vi "DAQLinescan.vi"() -> ()   [LabVIEW 2009]
uses:
  ImageSettings.ctt
  DisplaySettings.ctt
  Instance          51 19Saved   DAQLinescan .vi
  Instance          52 19Saved   DAQLinescan .vi
  <vilib>/Utility/inputDevices.llb/mouseAcquire.vi
  AO Update Channel.vi
panel:
  out "Position":dbl[](array[numeric]) format="%.6f"
  in  "show position (PI digital)":bool
  in  "mouse wheel\nfocus control":bool
  out "mouse focus":cluster{"device ID":refnum<k1>, "Scrolling":i32}
  in  "Laser 4":bool
  in  "SyncTime(ns)":dbl=12.5
  in  "Laser 3":bool
  in  "Laser 2":bool
  in  "Laser 1":bool
  in  "AOTF":u16(ring) items=["None", "Laser 1", "Laser 2", "Laser 1 + 2", "Laser 3", "Laser 1 + 3", "Laser 2 + 3", "Laser 1+2+3", "Laser 1+2+3+4", "Laser 2+3+4"]
  in  "AOTF Setup":bool
  in  "x-scale: Time?":bool
  in  "Autoscale y-axis":bool=TRUE
  in  "Store Data":bool
  in  "Pick & Destroy":bool caption="stop"
  in  "Load Image":bool caption="stop"
  in  "Position Increment (µm)":cluster{"x":dbl, "y":dbl, "z":dbl}={"x"=0.1, "y"=0.1, "z"=0.1} {"z" format="%.2f"; "y" format="%.2f"; "x" format="%.2f"}
  in  "Current Position (µm)":cluster{"x":dbl, "y":dbl, "z":dbl} {"z" format="%.2f"; "y" format="%.2f"; "x" format="%.2f"}
  in  "Down (z)":bool
  in  "Up (z)":bool
  in  "Down":bool
  in  "Up":bool
  in  "Right":bool
  in  "Left":bool
  in  "Display Settings":T1={"Show MCS"=TRUE, "Show Image"=TRUE, "Color coding"=1, "Plane"=0, "Threshold"={"max"=150, "min"=0}} {"Plane" max=0; "Color coding" items=["Color Gradient", "False Color"]}
  in  "Destination:":path
  in  "Exit":bool caption="stop"
  in  "Save & Exit":bool caption="stop"
  in  "Stage Setup":bool
  in  "SPC Setup":bool
  in  "Scan":bool
  in  "EOM Setup":bool
  in  "Keep Start Position":bool=TRUE
  in  "Isotropy (x/y)":bool=TRUE
  in  "Keep Image Size":bool=TRUE
  in  "EOM":u16(ring) items=["None", "Trace", "Retrace", "All"]
  in  "Read Position":bool
  in  "Image Settings":T2={"Start Position (µm)"={"x"=0.0, "y"=0.0, "z"=0.0}, "End Position (µm)"={"x"=10.0, "y"=10.0, "z"=10.0}, "Image Resolution (nm/pixel)"={"x"=50.0, "y"=50.0, "z"=100.0}, "Image Size (µm)"={"x"=10.0, "y"=10.0, "z"=0.0}, "Image Size (pixel)"={"x"=200, "y"=200, "z"=0}, "Time Resolution\n(ms/pixel)"=1.0, "1st Axis"=0, "2nd Axis"=1, "Retrace"=FALSE, "Estimated Time"="00:00:40"} {"2nd Axis" items=["x", "y", "z"]; "1st Axis" items=["x", "y", "z"]; "Time Resolution\n(ms/pixel)" format="%.2f"; "Image Resolution (nm/pixel)"."z" format="%.2f"; "Image Resolution (nm/pixel)"."y" format="%.2f"; "Image Resolution (nm/pixel)"."x" format="%.2f"; "Image Size (µm)"."z" format="%.2f"; "Image Size (µm)"."y" format="%.2f"; "Image Size (µm)"."x" format="%.2f"; "End Position (µm)"."z" format="%.2f"; "End Position (µm)"."y" format="%.2f"; "End Position (µm)"."x" format="%.2f"; "Start Position (µm)"."z" format="%.2f"; "Start Position (µm)"."y" format="%.2f"; "Start Position (µm)"."x" format="%.2f"}
  out "MCS Trace":u32[][](graph)=[[5, 9, 9, 4, 5, 7, 7, 7, 4, 6, 5, 11, 11, 6, 8, 9, 8, 5, 6, 8, 5, 5, 8, 5, 6, 5, 4, 9, 6, 13, 5, 5, 6, 9, 9, 11, 9, 7, 5, 9, 10, 7, 6, 4, 9, 7, 8, 6, 9, 4, 7, 9, 3, 4, 6, 8, 5, 6, 5, 4, 6, 11, 8, 5, 9, 5, 8, 7, 8, 8, 7, 3, 5, 14, 7, 12, 10, 7, 8, 8, 7, 5, 6, 6, 6, 9, 9, 7, 8, 7, 9, 3, 11, 4, 8, 7, 4, 4, 4, 5, 6, 6, 12, 5, 8, 7, 8, 7, 5, 8, 10, 10, 9, 5, 7, 8, 4, 6, 9, 6, 8, 9, 9, 9, 3, 7, 4, 10, 8, 11, 8, 6, 7, 4, 6, 4, 11, 9, 11, 7, 8, 4, 6, 9, 11, 8, 11, 7, 6, 4, 13, 9, 5, 4, 8, 5, 11, 5, 6, 6, 6, 3, 8, 8, 8, 11, 8, 6, 5, 7, 10, 7, 10, 12, 6, 9, 7, 4, 8, 8, 9, 7, 6, 6, 5, 8, 8, 3, 10, 5, 5, 7, 9, 8, 14, 6, 9, 5, 8, 7], [0, 0, 0, 0, 0, 0, 0, 0, 0, 0, 0, 0, 0, 0, 0, 0, 0, 0, 0, 0, 0, 0, 0, 0, 0, 0, 0, 0, 0, 0, 0, 0, 0, 0, 0, 0, 0, 0, 0, 0, 0, 0, 0, 0, 0, 0, 0, 0, 0, 0, 0, 0, 0, 0, 0, 0, 0, 0, 0, 0, 0, 0, 0, 0, 0, 0, 0, 0, 0, 0, 0, 0, 0, 0, 0, 0, 0, 0, 0, 0, 0, 0, 0, 0, 0, 0, 0, 0, 0, 0, 0, 0, 0, 0, 0, 0, 0, 0, 0, 0, 0, 0, 0, 0, 0, 0, 0, 0, 0, 0, 0, 0, 0, 0, 0, 0, 0, 0, 0, 0, 0, 0, 0, 0, 0, 0, 0, 0, 0, 0, 0, 0, 0, 0, 0, 0, 0, 0, 0, 0, 0, 0, 0, 0, 0, 0, 0, 0, 0, 0, 0, 0, 0, 0, 0, 0, 0, 0, 0, 0, 0, 0, 0, 0, 0, 0, 0, 0, 0, 0, 0, 0, 0, 0, 0, 0, 0, 0, 0, 0, 0, 0, 0, 0, 0, 0, 0, 0, 0, 0, 0, 0, 0, 0, 0, 0, 0, 0, 0, 0], [0, 0, 0, 0, 0, 0, 0, 0, 0, 0, 0, 0, 0, 0, 0, 0, 0, 0, 0, 0, 0, 0, 0, 0, 0, 0, 0, 0, 0, 0, 0, 0, 0, 0, 0, 0, 0, 0, 0, 0, 0, 0, 0, 0, 0, 0, 0, 0, 0, 0, 0, 0, 0, 0, 0, 0, 0, 0, 0, 0, 0, 0, 0, 0, 0, 0, 0, 0, 0, 0, 0, 0, 0, 0, 0, 0, 0, 0, 0, 0, 0, 0, 0, 0, 0, 0, 0, 0, 0, 0, 0, 0, 0, 0, 0, 0, 0, 0, 0, 0, 0, 0, 0, 0, 0, 0, 0, 0, 0, 0, 0, 0, 0, 0, 0, 0, 0, 0, 0, 0, 0, 0, 0, 0, 0, 0, 0, 0, 0, 0, 0, 0, 0, 0, 0, 0, 0, 0, 0, 0, 0, 0, 0, 0, 0, 0, 0, 0, 0, 0, 0, 0, 0, 0, 0, 0, 0, 0, 0, 0, 0, 0, 0, 0, 0, 0, 0, 0, 0, 0, 0, 0, 0, 0, 0, 0, 0, 0, 0, 0, 0, 0, 0, 0, 0, 0, 0, 0, 0, 0, 0, 0, 0, 0, 0, 0, 0, 0, 0, 0]]
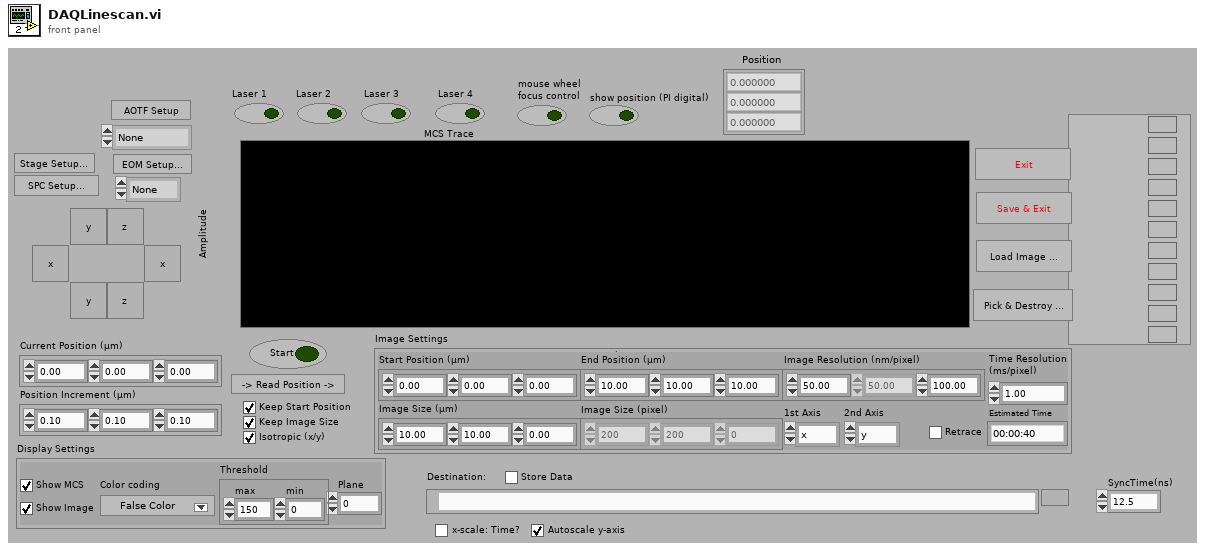
[diagram p1: front panel]
types:
  T1 = typedef "DisplaySettings.ctt" = cluster{"Show MCS":bool, "Show Image":bool, "Color coding":u16, "Plane":u32, "Threshold":cluster{"max":u32, "min":u32}}
  T2 = typedef "ImageSettings.ctt" = cluster{"Start Position (µm)":cluster{"x":dbl, "y":dbl, "z":dbl}, "End Position (µm)":cluster{"x":dbl, "y":dbl, "z":dbl}, "Image Resolution (nm/pixel)":cluster{"x":dbl, "y":dbl, "z":dbl}, "Image Size (µm)":cluster{"x":dbl, "y":dbl, "z":dbl}, "Image Size (pixel)":cluster{"x":u32, "y":u32, "z":u32}, "Time Resolution\n(ms/pixel)":dbl, "1st Axis":u16, "2nd Axis":u16, "Retrace":bool, "Estimated Time":string}
  T3 = enum16{"Get Type", "Set Type", "GetStageInit", "GetWriteStageSetting", "GetInitializeStageOutput", "GetSetAxisPosition", "GetSetPos", "GetSetupStage", "HaltStageOutput"}
  T4 = enum16{"Get Type", "Set Type", "GetStageInit", "GetWriteStageSetting", "GetInitializeStageOutput", "GetSetAxisPosition", "GetSetPos"}
  T5 = typedef "FIFOSettings.ctt" = cluster{"Measurement":cluster{"Binning (ms)":sgl, "External Trigger Condition":u16, "Stop Condition:":u16, "Stop Count":dbl, "Buffer Size (Photons)":u32, "No of Channels":u16, "Ext Latch Delay":i16}, "ADC":cluster{"Binning (HH)":i16, "Dither Range":i16, "Count Increment":i16, "Mode":u16}, "SYNC":cluster{"SYNC ZC Level (mV)":sgl, "SYNC Freq Divider":u16, "SYNC Holdoff (ps)":sgl, "SYNC Threshold (mV)":sgl}, "TAC":cluster{"TAC Range (ns)":sgl, "TAC Gain":i16, "TAC Offset (%)":sgl, "TAC Limit Low (%)":sgl, "TAC Limit High (%)":sgl}, "Ch 2":cluster{"Ch2 ZC Level (mV)":sgl, "Ch2 Holdoff (ps)":sgl, "Ch2 Threshold (mV)":sgl}, "Ch 3":cluster{"Ch3 ZC Level (mV)":sgl, "Ch3 Holdoff (ps)":sgl, "Ch3 Threshold (mV)":sgl}, "Ch 4":cluster{"Ch4 ZC Level (mV)":sgl, "Ch4 Holdoff (ps)":sgl, "Ch4 Threshold (mV)":sgl}, "Ch1":cluster{"Ch1 ZC Level (mV)":sgl, "Ch1 Holdoff (ps)":sgl, "Ch1 Threshold (mV)":sgl}}
  T6 = typedef "DAQLinescanVisualization.ctt" = cluster{"Threshold":u32, "Trace Window #":u32, "IMAQ Trace":T7, "Retrace Window #":u32, "IMAQ Retrace":T7}
  T7 = typedef "IMAQ Image.ctl" = refnum<image>
  T8 = typedef "LineScanStatus.ctt" = cluster{"in line":bool, "line status":cluster{"count":u32, "current":cluster{"x":u32, "y":u32, "z":u32}}, "plane status":cluster{"count":u32, "current":cluster{"x":u32, "y":u32, "z":u32}}, "new line step":cluster{"x":dbl, "y":dbl, "z":dbl}, "new plane step":cluster{"x":dbl, "y":dbl, "z":dbl}}
  T9 = typedef "StageType.ctt" = enum16{"PI analogue", "PI 712 TCP/IP", "Märzhäuser", "PI analogue step", "PI 712 USB"}
  T10 = cluster{"Start Position (µm)":cluster{"x":dbl, "y":dbl, "z":dbl}, "End Position (µm)":cluster{"x":dbl, "y":dbl, "z":dbl}, "Image Resolution (nm/pixel)":cluster{"x":dbl, "y":dbl, "z":dbl}, "Image Size (µm)":cluster{"x":dbl, "y":dbl, "z":dbl}, "Image Size (pixel)":cluster{"x":u32, "y":u32, "z":u32}, "Time Resolution\n(ms/pixel)":dbl, "1st Axis":u16, "2nd Axis":u16, "Retrace":bool, "Estimated Time":string}
  T11 = typedef "ScannedImage.ctl" = cluster{"BinningMicroS":dbl, "OverflowConstant":dbl, "MacrotimeCycle":dbl, "Trace":u32[][][][], "Retrace":u32[][][][], "current line":i32, "current plane":i32}
  T12 = cluster{"Horizontal":i32, "Vertical":i32, "Scrolling":i32}
  T13 = typedef "LVMinMaxIncTypeDef.ctl" = cluster{"Minimum":dbl, "Maximum":dbl, "Increment":dbl}
  T14 = typedef "AnalogSettings.ctt" = cluster{"PCI 671x Device Number":u32, "Samples per Unit":u32}
  T15 = typedef "AOTFSettings.ctt" = cluster{"Laser 1 Output Channel":tag, "AOTF  1 Output Voltage":dbl, "Laser 2 Output Channel":tag, "AOTF  2 Output Voltage":dbl, "Laser 3 Output Channel":tag, "AOTF  3 Output Voltage":dbl, "Pixel per Cycle":u16, "Time per Cycle  / ms":dbl, "Laser 4 Output Channel":tag, "AOTF  4 Output Voltage":dbl}
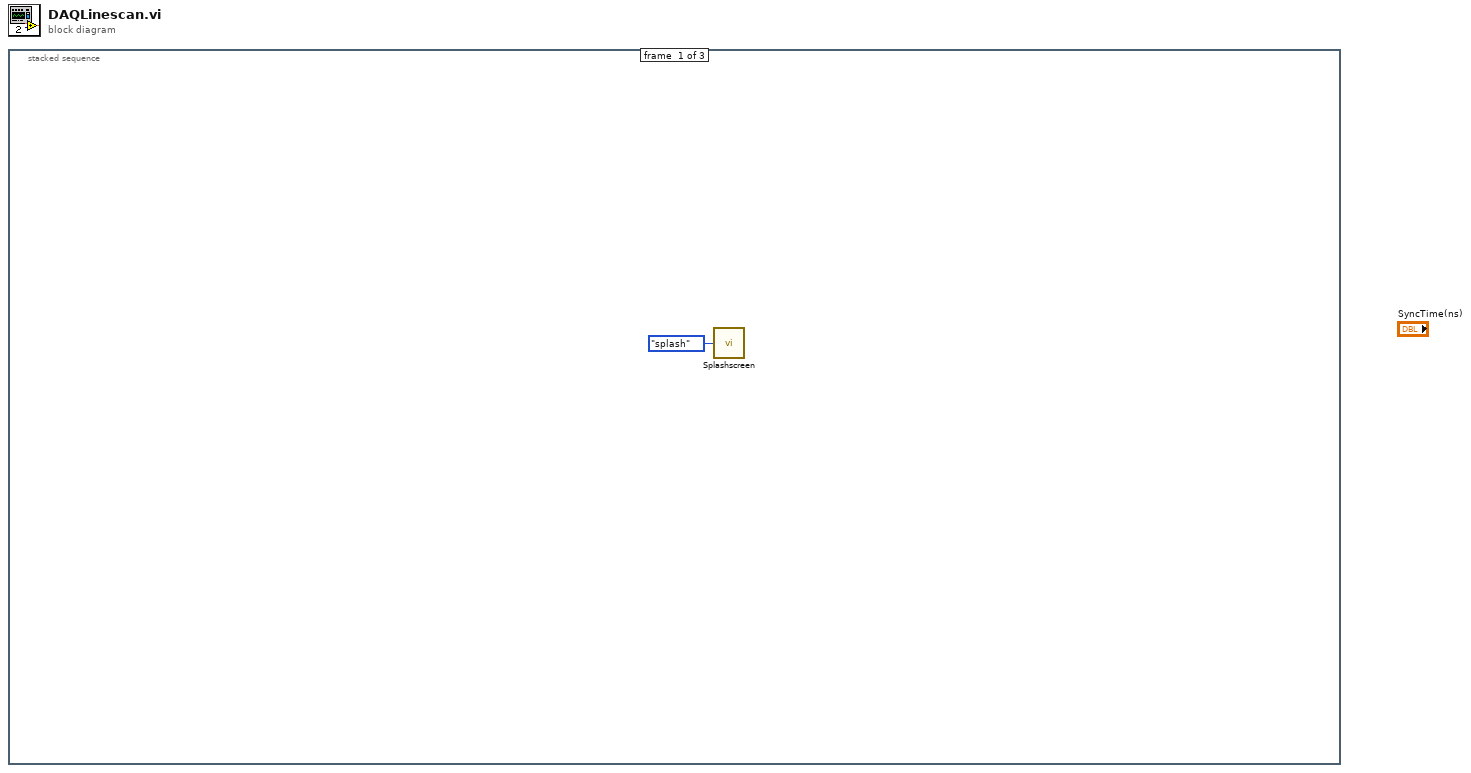
[diagram p0: block diagram]
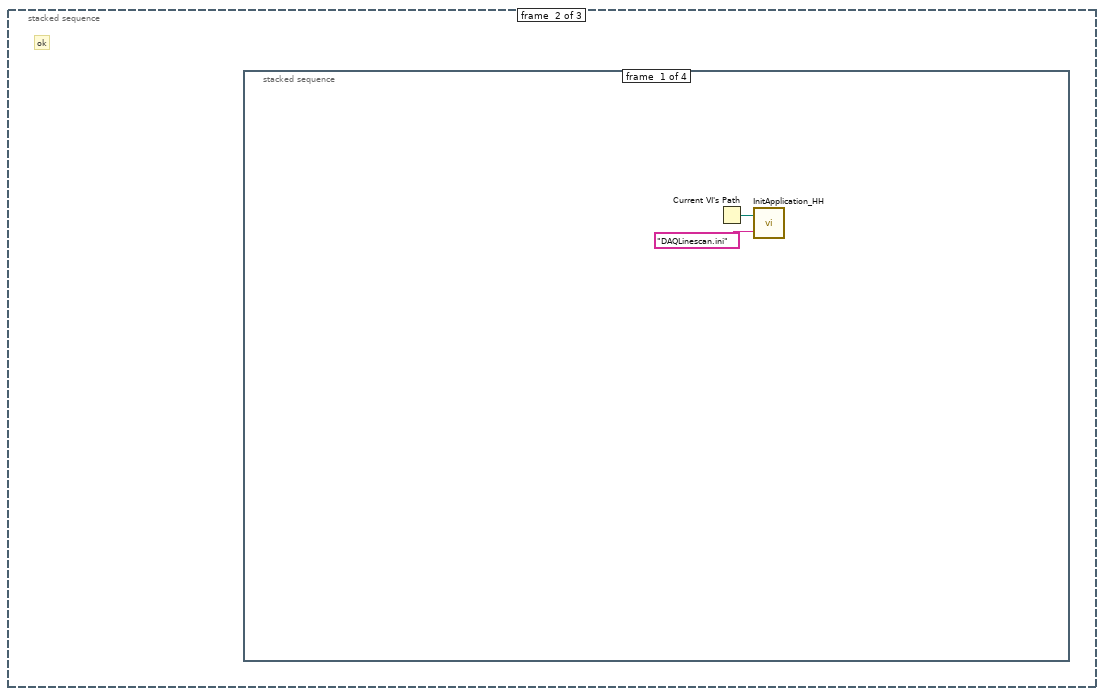
[diagram p2: hidden frame]
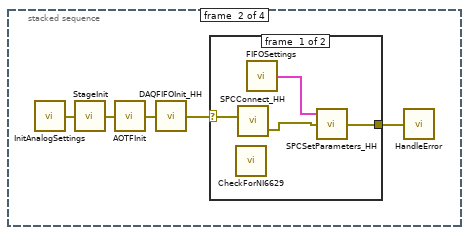
[diagram p3: hidden frame]
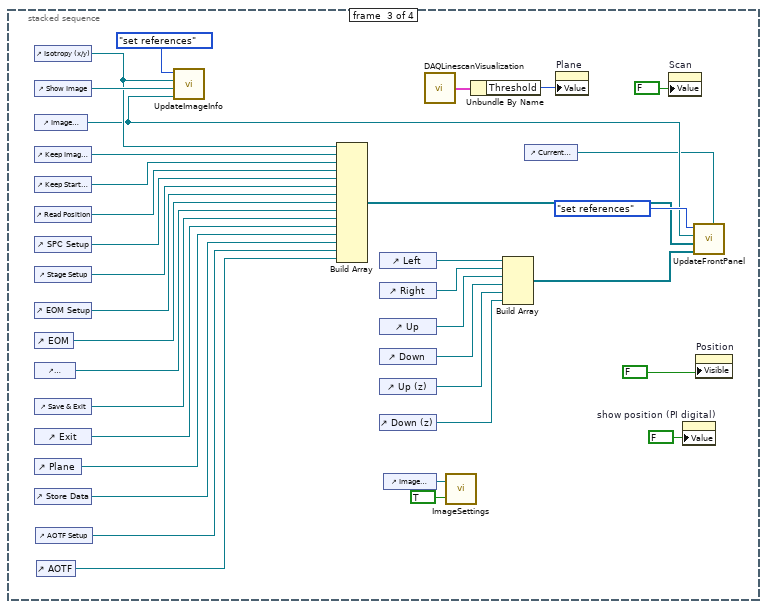
[diagram p5: hidden frame]
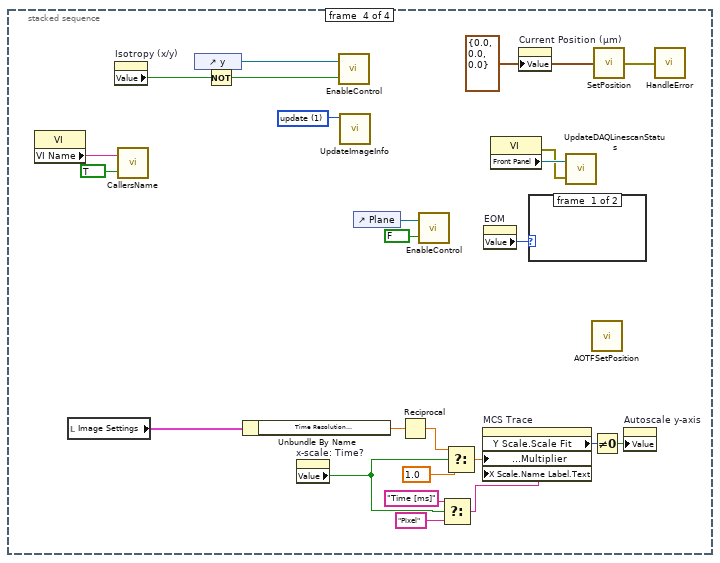
[diagram p6: hidden frame]
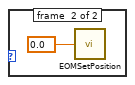
[diagram p7: hidden frame]
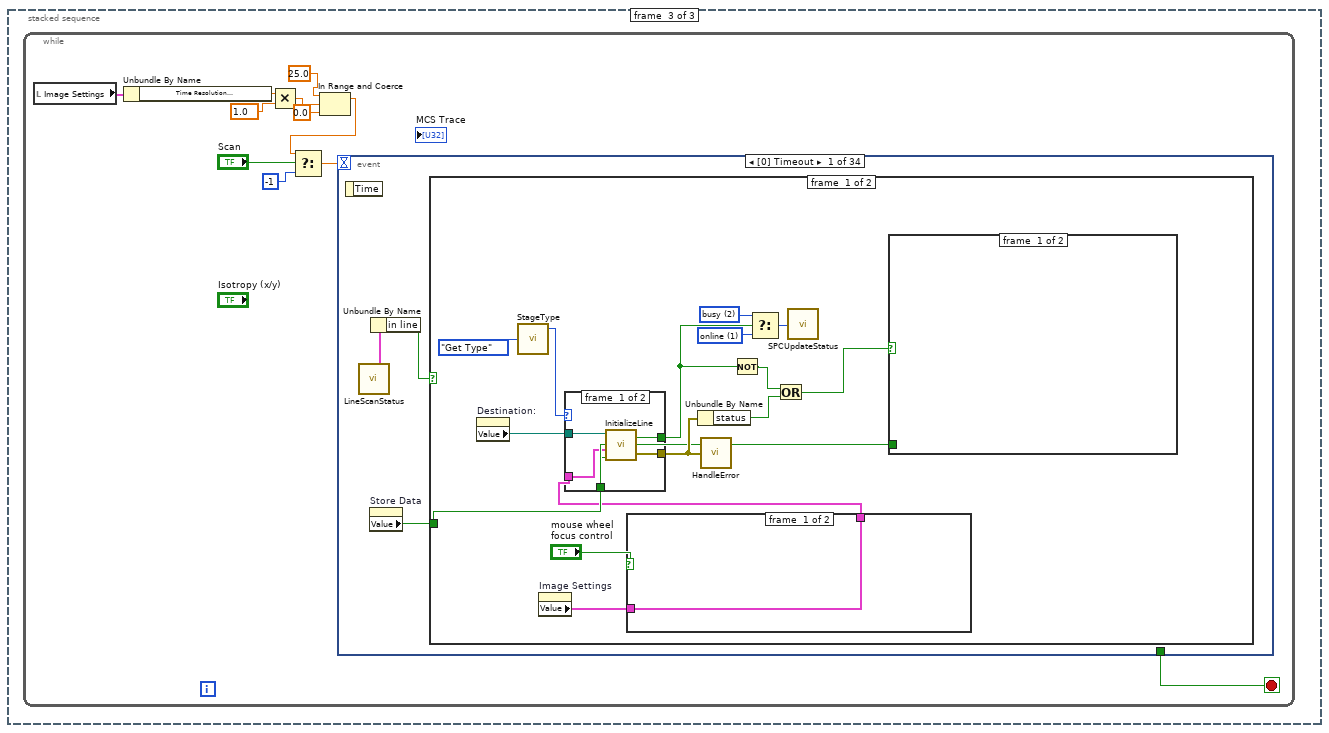
[diagram p8: hidden frame]
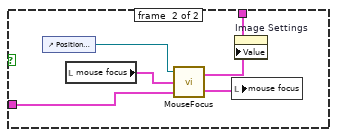
[diagram p9: hidden frame]
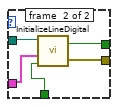
[diagram p10: hidden frame]
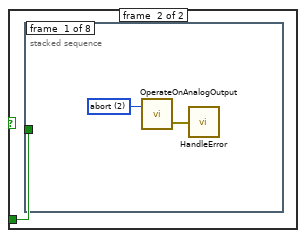
[diagram p11: hidden frame]
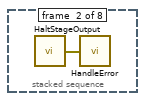
[diagram p12: hidden frame]
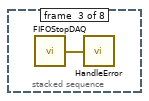
[diagram p13: hidden frame]
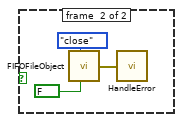
[diagram p15: hidden frame]
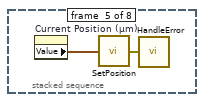
[diagram p16: hidden frame]
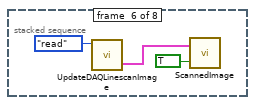
[diagram p17: hidden frame]
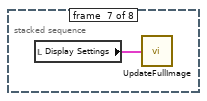
[diagram p18: hidden frame]
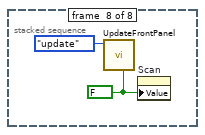
[diagram p19: hidden frame]
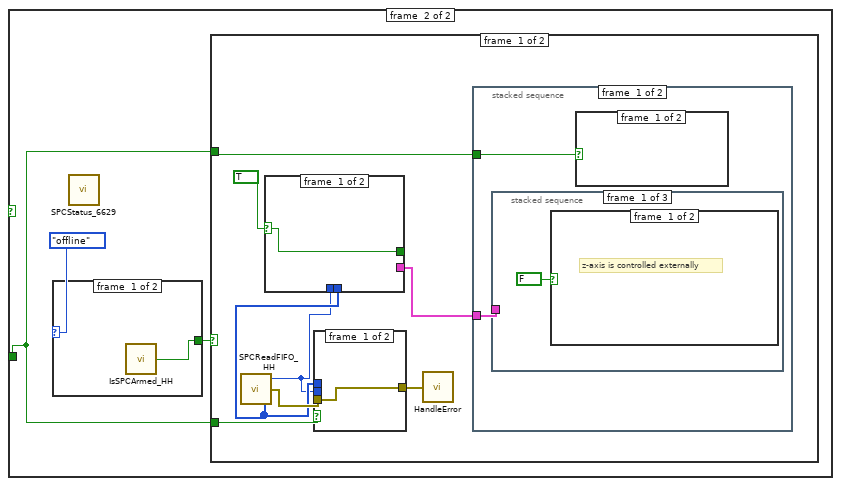
[diagram p20: hidden frame]
diagram:
  n1 = stacked-sequence {
    frame #0 {
      n2 = call "Splashscreen.vi"("Mode"=enum16{"splash", "dialog"}."splash") -> ()  [unwired: 1 in]
    }
    frame #1 {
      # "ok"
      n3 = stacked-sequence {
        frame #0 {
          n4 = Current VI's Path() -> (path=w3:path)
          n5 = call "InitApplication_HH.vi"("file name"="DAQLinescan.ini", "VI path"=w3) -> ()
        }
        frame #1 {
          n6 = call "InitAnalogSettings.vi"() -> ("error out"=w5:errorcluster)  [unwired: 1 in]
          n7 = call "StageInit.vi"("error in (no error)"=w5) -> ("error out"=w4:errorcluster)
          n8 = call "AOTFInit.vi"("error in (no error)"=w4) -> ("error out"=w6:errorcluster)
          n9 = call "DAQFIFOInit_HH.vi"("error in (no error)"=w6) -> ("error out"=w8:errorcluster)
          n10 = case shown="No Error" w8 {
            selector: w8 -> [w10 w13]
            tunnel: [w11 w13] -> w7
            frame #0 {
              n11 = call "CheckForNI6629.vi"() -> ()  [unwired: 1 in]
              n12 = call "SPCConnect_HH.vi"("error in (no error)"=w10) -> ("Error out"=w9:errorcluster)  [unwired: 1 in]
              n13 = call "FIFOSettings.vi"() -> ("FIFO Settings(out)"=w12:T5)  [unwired: 2 in]
              n14 = call "SPCSetParameters_HH.vi"("error in (no error)"=w9, "FIFO Settings"=w12) -> ("error (out)"=w11:errorcluster)  [unwired: 1 in]
            }
            frame #1 {
            }
          }
          n15 = call "HandleError.vi"("error in (no error)"=w7) -> ()
        }
        frame #2 {
          n16 = control-ref of="Isotropy (x/y)"() -> (w27:refnum<vi>)
          n17 = control-ref of="Show Image"() -> (w46:refnum<vi>)
          n18 = control-ref of="Image Settings"() -> (w26:refnum<vi>)
          n19 = control-ref of="Keep Image Size"() -> (w45:refnum<vi>)
          n20 = control-ref of="Keep Start Position"() -> (w44:refnum<vi>)
          n21 = control-ref of="Read Position"() -> (w43:refnum<vi>)
          n22 = control-ref of="SPC Setup"() -> (w42:refnum<vi>)
          n23 = control-ref of="Stage Setup"() -> (w41:refnum<vi>)
          n24 = control-ref of="EOM Setup"() -> (w40:refnum<vi>)
          n25 = control-ref of="EOM"() -> (w39:refnum<vi>)
          n26 = control-ref of="Destination:"() -> (w38:refnum<vi>)
          n27 = control-ref of="Save & Exit"() -> (w37:refnum<vi>)
          n28 = control-ref of="Exit"() -> (w36:refnum<vi>)
          n29 = control-ref of="Plane"() -> (w22:refnum<vi>)
          n30 = control-ref of="Store Data"() -> (w21:refnum<vi>)
          n31 = control-ref of="AOTF Setup"() -> (w17:refnum<vi>)
          n32 = control-ref of="AOTF"() -> (w16:refnum<vi>)
          n33 = call "UpdateImageInfo.vi"("Image Refnum"=w26, "Show Image Refnum"=w46, "Isotropy (x/y) Refnum"=w27, "operation"=enum16{"set references", "update"}."set references") -> ()
          n34 = Build Array(w27, w45, w44, w43, w42, w41, w40, w39, w38, w37, w36, w22, w21, w17, w16) -> (w25:refnum<vi>[])
          n35 = control-ref of="Left"() -> (w35:refnum<vi>)
          n36 = control-ref of="Right"() -> (w34:refnum<vi>)
          n37 = control-ref of="Up"() -> (w33:refnum<vi>)
          n38 = control-ref of="Down"() -> (w32:refnum<vi>)
          n39 = control-ref of="Up (z)"() -> (w31:refnum<vi>)
          n40 = control-ref of="Down (z)"() -> (w30:refnum<vi>)
          n41 = control-ref of="Image Settings"() -> (w19:refnum<vi>)
          n42 = call "DAQLinescanVisualization.vi"() -> ("Visualization (output)"=w47:T6)  [unwired: 2 in]
          n43 = call "ImageSettings.vi"("set"=TRUE ("s"), "Image Settings in"=w19) -> ()  [unwired: 1 out]
          n44 = Unbundle By Name(w47) -> ("Threshold"=w48:u32)
          n45 = Build Array(w35, w34, w33, w32, w31, w30) -> (w24:refnum<vi>[])
          n46 = control-ref of="Current Position (µm)"() -> (w23:refnum<vi>)
          n47 = property on="Plane" class="DigNum (strict)"("Value"=w48) -> ()  [unwired: 2 in, 2 out]
          n48 = property on="Scan" class="Bool (strict)"("Value"=FALSE ("Scan")) -> ()  [unwired: 2 in, 2 out]
          n49 = property on="show position (PI digital)" class="Bool (strict)"("Value"=FALSE ("show position (PI digital)")) -> ()  [unwired: 2 in, 2 out]
          n50 = call "UpdateFrontPanel.vi"("operation"=enum16{"set references", "update"}."set references", "Image Settings"=w26, "Regular Controls"=w25, "Special Controls"=w24, "Current Position (µm)"=w23) -> ()  [unwired: 5 in]
          n51 = property on="Position" class="Arr (strict)"("Visible"=FALSE) -> ()  [unwired: 2 in, 2 out]
        }
        frame #3 {
          w66 = u16 1 items=["set references", "update"] ("operation")
          w70 = cluster{"x":dbl, "y":dbl, "z":dbl} {"x"=0.0, "y"=0.0, "z"=0.0} ("Current Position (µm)")
          n52 = property class="VI"() -> ("VI Name"=w61:string)  [unwired: 2 in, 2 out]
          n53 = local read "Image Settings"() -> (w57:T2)
          n54 = property on="Isotropy (x/y)" class="Boolean (strict)"() -> ("Value"=w67:bool)  [unwired: 2 in, 2 out]
          n55 = call "CallersName.vi"("Get/Set"=TRUE ("s"), "Callers Name"=w61) -> ()  [unwired: 1 out]
          n56 = control-ref of="y"() -> (w72:refnum<vi>)
          n57 = Not(x=w67) -> (.not. x?=w71:bool)
          n58 = Unbundle By Name(w57) -> ("Time Resolution\n(ms/pixel)"=w56:dbl)
          n59 = property on="x-scale: Time?" class="Boolean (strict)"() -> ("Value"=w50:bool)  [unwired: 2 in, 2 out]
          n60 = call "EnableControl.vi"("Enable"=w71, "Reference"=w72) -> ()
          n61 = call "UpdateImageInfo.vi"("operation"=w66) -> ()  [unwired: 3 in]
          n62 = control-ref of="Plane"() -> (w65:refnum<vi>)
          n63 = Reciprocal(x=w56) -> (1/x=w54:dbl)
          n64 = call "EnableControl.vi"("Enable"=FALSE, "Reference"=w65) -> ()
          n65 = Select(t="Time [ms]", s=w50, f="Pixel") -> (s? t:f=w49:string)
          n66 = Select(t=w54, s=w50, f=1.0) -> (s? t:f=w55:dbl)
          n67 = property on="MCS Trace" class="WaveformChart (strict)"("X Scale.Offset and Multiplier:Multiplier"=w55, "X Scale.Name Label.Text"=w49) -> ("Y Scale.Scale Fit"=w59:u8)  [unwired: 2 in, 2 out]
          n68 = property on="EOM" class="Ring (strict)"() -> ("Value"=w62:u16)  [unwired: 2 in, 2 out]
          n69 = property class="VI"() -> (error out=w68:errorcluster, "Front Panel"=w69:refnum<vi>)  [unwired: 2 in, 1 out]
          n70 = property on="Current Position (µm)" class="Cluster (strict)"("Value"=w70) -> ()  [unwired: 2 in, 2 out]
          n71 = case shown="0" w62 {
            frame #0 {
            }
            frame #1 {
              n72 = call "EOMSetPosition.vi"("value"=sgl 0.0) -> ()
            }
          }
          n73 = call "UpdateDAQLinescanStatus.vi"("error in (no error)"=w68, "Panel"=w69) -> ()
          n74 = call "AOTFSetPosition.vi"() -> ()  [unwired: 2 in]
          n75 = Not Equal To 0?(x=w59) -> (x != 0?=w58:bool)
          n76 = call "SetPosition.vi"("Current Position (µm)"=w70) -> ("error out"=w63:errorcluster)
          n77 = property on="Autoscale y-axis" class="Bool (strict)"("Value"=w58) -> ()  [unwired: 2 in, 2 out]
          n78 = call "HandleError.vi"("error in (no error)"=w63) -> ()
        }
      }
    }
    frame #2 {
      n79 = while {
        stop <- w80 stop-if-true
        n80 = local read "Image Settings"() -> (w81:T2)
        n81 = Unbundle By Name(w81) -> ("Time Resolution\n(ms/pixel)"=w79:dbl)
        n82 = Multiply(x=w79, y=1.0) -> (x*y=w77:dbl)
        n83 = In Range and Coerce(upper limit=25.0, x=w77, lower limit=0.0) -> (coerced(x)=w74:dbl)  [unwired: 1 out]
        n84 = Select(t=w74, s="Scan", f=-1) -> (s? t:f=w84:dbl)
        n85 = event shown="[0] Timeout" {
          selector: _ -> [_ _ _ _ _ _ _ _ _ _ _ _ _ _ _ _ _ _ _ _ _ _ _ _ _ _ _ _ _ _ _ _ _ _]
          dyn-events: _ -> [_ _ _ _ _ _ _ _ _ _ _ _ _ _ _ _ _ _ _ _ _ _ _ _ _ _ _ _ _ _ _ _ _ _]
          timeout: w84 -> [_ _ _ _ _ _ _ _ _ _ _ _ _ _ _ _ _ _ _ _ _ _ _ _ _ _ _ _ _ _ _ _ _ _]
          tunnel: [_ _ _ _ _ _ _ _ _ _ _ _ _ _ _ _ _ _ _ _ _ _ _ _ _ TRUE _ _ _ _ _ _ _ _] -> w80
          event #0 {
            n86 = event-data() -> ()  [unwired: 1 in, 1 out]
            n87 = call "LineScanStatus.vi"() -> ("Linescan Status (output)"=w86:T8)  [unwired: 2 in]
            n88 = property on="Store Data" class="Boolean (strict)"() -> ("Value"=w85:bool)  [unwired: 2 in, 2 out]
            n89 = Unbundle By Name(w86) -> ("in line"=w87:bool)
            n90 = case shown="True" w87 {
              tunnel: w85 -> [w93 w138]
              frame #0 {
                w100 = u16 1 items=["offline", "online", "busy"] ("Status (input)")
                w101 = u16 2 items=["offline", "online", "busy"] ("Status (input)")
                n91 = property on="Destination:" class="Path"() -> ("Value"=w102:path)  [unwired: 2 in, 2 out]
                n92 = call "StageType.vi"("Function"=T3."Get Type") -> ("Stage Type (output)"=w91:T9)  [unwired: 2 in, 2 out]
                n93 = property on="Image Settings" class="Cluster (strict)"() -> ("Value"=w90:T10)  [unwired: 2 in, 2 out]
                n94 = case shown="False" "mouse wheel\nfocus control" {
                  tunnel: w90 -> [w103 w108]
                  tunnel: [w103 w107] -> w89
                  frame #0 {
                  }
                  frame #1 {
                    n95 = control-ref of="Position Increment (µm)"() -> (w104:refnum<vi>)
                    n96 = local read "mouse focus"() -> (w106:cluster{"device ID":refnum<k1>, "Scrolling":i32})
                    n97 = call "MouseFocus.vi"("Image Settings"=w108, "mouse focus"=w106, "Position increment"=w104) -> ("mouse focus"=w105:cluster{"device ID":refnum<k1>, "Scrolling":i32}, "Image Settings"=w107:T10)
                    n98 = local write "mouse focus"(w105) -> ()
                    n99 = property on="Image Settings" class="Clust (strict)"("Value"=w107) -> ()  [unwired: 2 in, 2 out]
                  }
                }
                n100 = case shown="\"PI 712 TCP/IP\", \"PI 712 USB\"" w91 {
                  tunnel: w102 -> [w113 w118]
                  tunnel: w89 -> [w112 w117]
                  tunnel: [w111 w115] -> w98
                  tunnel: [w110 w114] -> w97
                  tunnel: w93 -> [w109 w116]
                  frame #0 {
                    n101 = call "InitializeLine.vi"("Store Data"=w109, "Image Settings"=w112, "Destination:"=w113) -> ("error out"=w111:errorcluster, "Busy"=w110:bool)  [unwired: 1 in]
                  }
                  frame #1 {
                    n102 = call "InitializeLineDigital.vi"("Store Data"=w116, "Image Settings"=w117, "Destination:"=w118) -> ("error out"=w115:errorcluster, "Busy"=w114:bool)  [unwired: 1 in]
                  }
                }
                n103 = Unbundle By Name(w98) -> ("status"=w95:bool)
                n104 = call "HandleError.vi"("error in (no error)"=w98) -> ()
                n105 = Not(x=w97) -> (.not. x?=w96:bool)
                n106 = Select(t=w101, s=w97, f=w100) -> (s? t:f=w99:u16)
                n107 = Or(x=w96, y=w95) -> (x .or. y?=w94:bool)
                n108 = call "SPCUpdateStatus.vi"("Status"=w99) -> ()
                n109 = case shown="False" w94 {
                  tunnel: w93 -> [_ w119]
                  frame #0 {
                  }
                  frame #1 {
                    n110 = stacked-sequence {
                      tunnel: w119 -> [_ _ _ w124 _ _ _ _]
                      frame #0 {
                        w121 = u16 2 items=["start", "state", "abort"] ("operation")
                        n111 = call "OperateOnAnalogOutput.vi"("operation"=w121) -> ("error out"=w120:errorcluster)  [unwired: 1 in, 1 out]
                        n112 = call "HandleError.vi"("error in (no error)"=w120) -> ()
                      }
                      frame #1 {
                        n113 = call "HaltStageOutput.vi"() -> ("Error out"=w122:errorcluster)  [unwired: 1 in]
                        n114 = call "HandleError.vi"("error in (no error)"=w122) -> ()
                      }
                      frame #2 {
                        n115 = call "FIFOStopDAQ.vi"() -> ("error out"=w123:errorcluster)
                        n116 = call "HandleError.vi"("error in (no error)"=w123) -> ()
                      }
                      frame #3 {
                        n117 = case shown="True" w124 {
                          frame #0 {
                          }
                          frame #1 {
                            n118 = call "FIFOFileObject.vi"(".sm file format"=FALSE, "function (open:0)"=enum16{"open", "write", "close"}."close") -> ("error out"=w126:errorcluster)  [unwired: 4 in]
                            n119 = call "HandleError.vi"("error in (no error)"=w126) -> ()
                          }
                        }
                      }
                      frame #4 {
                        n120 = property on="Current Position (µm)" class="Cluster (strict)"() -> ("Value"=w129:cluster{"x":dbl, "y":dbl, "z":dbl})  [unwired: 2 in, 2 out]
                        n121 = call "SetPosition.vi"("Current Position (µm)"=w129) -> ("error out"=w128:errorcluster)
                        n122 = call "HandleError.vi"("error in (no error)"=w128) -> ()
                      }
                      frame #5 {
                        n123 = call "UpdateDAQLinescanImage.vi"("operation"=enum16{"initialize", "update", "read"}."read") -> ("LinescanSampling"=w132:T11)  [unwired: 3 in, 1 out]
                        n124 = call "ScannedImage.vi"("Get/Set"=TRUE, "Scanned Image (input)"=w132) -> ()  [unwired: 1 out]
                      }
                      frame #6 {
                        n125 = local read "Display Settings"() -> (w133:T1)
                        n126 = call "UpdateFullImage.vi"("Display Settings"=w133) -> ()
                      }
                      frame #7 {
                        w135 = FALSE ("Scan")
                        n127 = call "UpdateFrontPanel.vi"("operation"=enum16{"set references", "update"}."update", "Scan"=w135) -> ()  [unwired: 8 in]
                        n128 = property on="Scan" class="Boolean (strict)"("Value"=w135) -> ()  [unwired: 2 in, 2 out]
                      }
                    }
                  }
                }
              }
              frame #1 {
                n129 = case shown="\"offline\", Default" enum16{"offline", "online", "busy"}."offline" ("Status (output)") {
                  tunnel: [w139 FALSE] -> w137
                  frame #0 {
                    n130 = call "IsSPCArmed_HH.vi"() -> ("Boolean"=w139:bool)  [unwired: 1 in]
                  }
                  frame #1 {
                  }
                }
                n131 = call "SPCStatus_6629.vi"() -> ()  [unwired: 2 in, 1 out]
                n132 = case shown="True" w137 {
                  tunnel: w138 -> [w141 w186]
                  tunnel: w138 -> [w143 w185]
                  frame #0 {
                    n133 = call "SPCReadFIFO_HH.vi"() -> ("count"=w144:i32, "error out"=w148:errorcluster, "buffer"=w146:u32[])  [unwired: 2 in]
                    n134 = case shown="True" TRUE ("Case Constant\n(See Context Help) 2") {
                      selector: TRUE ("Case Constant\n(See Context Help) 2") -> [w169 _]
                      tunnel: w144 -> [_ w174]
                      tunnel: w146 -> [_ w173]
                      tunnel: [w169 w172] -> _
                      tunnel: [_ w171] -> w142
                      frame #0 {
                      }
                      frame #1 {
                        n135 = call "UpdateDAQLinescanImage.vi"("buffer (output)"=w173, "count (read)"=w174, "operation"=enum16{"initialize", "update", "read"}."update") -> ("LinescanSampling"=w171:T11, "end of line"=w172:bool)  [unwired: 1 in]
                      }
                    }
                    n136 = case shown="True" w143 {
                      tunnel: w148 -> [w175 w180]
                      tunnel: [w175 w179] -> w147
                      tunnel: w144 -> [_ w178]
                      tunnel: w146 -> [_ w177]
                      frame #0 {
                      }
                      frame #1 {
                        n137 = call "FIFOFileObject.vi"(".sm file format"=FALSE, "function (open:0)"=enum16{"open", "write", "close"}."write", "error in (no error)"=w180, "count"=w178, "buffer"=w177) -> ("error out"=w179:errorcluster)  [unwired: 1 in]
                      }
                    }
                    n138 = call "HandleError.vi"("error in (no error)"=w147) -> ()
                    n139 = stacked-sequence {
                      tunnel: w142 -> [w150 _]
                      tunnel: w141 -> [w149 _]
                      frame #0 {
                        n140 = stacked-sequence {
                          tunnel: w150 -> [_ _ w160]
                          frame #0 {
                            n141 = case shown="True" FALSE {
                              frame #0 {
                                # "z-axis is controlled externally"
                              }
                              frame #1 {
                                w153 = 2
                                # "third axis"
                                n142 = property on="Current Position (µm)" class="Clust (strict)"() -> ("Value"=w152:cluster{"x":dbl, "y":dbl, "z":dbl})  [unwired: 2 in, 2 out]
                                n143 = Cluster To Array(cluster=w152) -> (array=w154:dbl[])
                                n144 = Index Array(array=w154, index=w153) -> (element=w155:dbl)
                                n145 = call "SetAxisPos.vi"("Position"=w155, "Axis"=w153) -> ("error out"=w156:errorcluster)
                                n146 = call "HandleError.vi"("error in (no error)"=w156) -> ()
                              }
                            }
                          }
                          frame #1 {
                            n147 = call "HaltStageOutput.vi"() -> ("Error out"=w157:errorcluster)  [unwired: 1 in]
                            n148 = call "HandleError.vi"("error in (no error)"=w157) -> ()
                          }
                          frame #2 {
                            n149 = call "FIFOStopDAQ.vi"() -> ("error out"=w161:errorcluster)
                            n150 = call "HandleError.vi"("error in (no error)"=w161) -> ()
                            n151 = call "OperateOnAnalogOutput.vi"("operation"=enum16{"start", "state", "abort"}."abort") -> ("error out"=w162:errorcluster)  [unwired: 1 in, 1 out]
                            n152 = call "UpdateDAQLinescanDisplay.vi"("LinescanSampling"=w160, "operation"=enum16{"initialize", "update"}."update") -> ()  [unwired: 3 in]
                            n153 = call "HandleError.vi"("error in (no error)"=w162) -> ()
                          }
                        }
                        n154 = case shown="True" w149 {
                          frame #0 {
                          }
                          frame #1 {
                            n155 = call "FIFOFileObject.vi"(".sm file format"=FALSE, "function (open:0)"=enum16{"open", "write", "close"}."close") -> ("error out"=w164:errorcluster)  [unwired: 4 in]
                            n156 = call "HandleError.vi"("error in (no error)"=w164) -> ()
                          }
                        }
                      }
                      frame #1 {
                        n157 = local read "Image Settings"() -> (w166:T2)
                        n158 = call "NextLine.vi"("Image Settings"=w166) -> ("Continue Scan"=w167:bool)
                        n159 = case shown="True" w167 {
                          frame #0 {
                          }
                          frame #1 {
                          }
                        }
                        n160 = call "UpdateFrontPanel.vi"("operation"=enum16{"set references", "update"}."update", "Scan"=w167) -> ()  [unwired: 8 in]
                        n161 = property on="Scan" class="Bool (strict)"("Value"=w167) -> ()  [unwired: 2 in, 2 out]
                      }
                    }
                  }
                  frame #1 {
                    n162 = call "SPCReadFIFO_HH.vi"() -> ("count"=w182:i32, "error out"=w190:errorcluster, "buffer"=w188:u32[])  [unwired: 2 in]
                    n163 = case shown="True" TRUE ("Case Constant\n(See Context Help) 2") {
                      selector: TRUE ("Case Constant\n(See Context Help) 2") -> [w191 _]
                      tunnel: w182 -> [_ w196]
                      tunnel: w188 -> [_ w195]
                      tunnel: [w191 w194] -> w183
                      tunnel: [_ w193] -> w187
                      frame #0 {
                      }
                      frame #1 {
                        n164 = call "UpdateDAQLinescanImage.vi"("buffer (output)"=w195, "count (read)"=w196, "operation"=enum16{"initialize", "update", "read"}."update") -> ("LinescanSampling"=w193:T11, "end of line"=w194:bool)  [unwired: 1 in]
                      }
                    }
                    n165 = case shown="False" w185 {
                      tunnel: w190 -> [w197 w202]
                      tunnel: [w197 w201] -> w189
                      tunnel: w182 -> [_ w200]
                      tunnel: w188 -> [_ w199]
                      frame #0 {
                      }
                      frame #1 {
                        n166 = call "FIFOFileObject.vi"(".sm file format"=FALSE, "function (open:0)"=enum16{"open", "write", "close"}."write", "error in (no error)"=w202, "count"=w200, "buffer"=w199) -> ("error out"=w201:errorcluster)  [unwired: 1 in]
                      }
                    }
                    n167 = call "HandleError.vi"("error in (no error)"=w189) -> ()
                    n168 = case shown="True" w183 {
                      tunnel: w187 -> [_ w205]
                      tunnel: w186 -> [_ w204]
                      frame #0 {
                      }
                      frame #1 {
                        n169 = stacked-sequence {
                          tunnel: w205 -> [w207 w229]
                          tunnel: w204 -> [w206 _]
                          frame #0 {
                            n170 = stacked-sequence {
                              tunnel: w207 -> [_ _ w218]
                              frame #0 {
                                w208 = 2
                                # "third axis"
                                n171 = property on="Current Position (µm)" class="Cluster (strict)"() -> ("Value"=w211:cluster{"x":dbl, "y":dbl, "z":dbl})  [unwired: 2 in, 2 out]
                                n172 = Cluster To Array(cluster=w211) -> (array=w209:dbl[])
                                n173 = Index Array(array=w209, index=w208) -> (element=w210:dbl)
                                n174 = call "SetAxisPos.vi"("Position"=w210, "Axis"=w208) -> ("error out"=w212:errorcluster)
                                n175 = call "HandleError.vi"("error in (no error)"=w212) -> ()
                              }
                              frame #1 {
                                n176 = call "HaltStageOutput.vi"() -> ("Error out"=w213:errorcluster)  [unwired: 1 in]
                                n177 = call "HandleError.vi"("error in (no error)"=w213) -> ()
                              }
                              frame #2 {
                                n178 = call "FIFOStopDAQ.vi"() -> ("error out"=w219:errorcluster)
                                n179 = call "StageType.vi"("Function"=T4."Get Type") -> ("Stage Type (output)"=w214:T9)  [unwired: 2 in, 2 out]
                                n180 = call "HandleError.vi"("error in (no error)"=w219) -> ()
                                n181 = case shown="\"PI 712 TCP/IP\"" w214 {
                                tunnel: [w222 w223] -> w220
                                tunnel: enum16{"start", "state", "abort"}."abort" ("operation") -> [w221 w224]
                                frame #0 {
                                n182 = call "OperateOnAnalogOutput.vi"("operation"=w221) -> ("error out"=w222:errorcluster)  [unwired: 1 in, 1 out]
                                }
                                frame #1 {
                                n183 = call "OperateOnDigitalOutput.vi"("operation"=w224) -> ("error out"=w223:errorcluster)  [unwired: 3 in]
                                }
                                }
                                n184 = call "UpdateDAQLinescanDisplay.vi"("LinescanSampling"=w218, "operation"=enum16{"initialize", "update"}."update") -> ()  [unwired: 3 in]
                                n185 = call "HandleError.vi"("error in (no error)"=w220) -> ()
                              }
                            }
                            n186 = case shown="False" w206 {
                              frame #0 {
                              }
                              frame #1 {
                                n187 = call "FIFOFileObject.vi"(".sm file format"=FALSE, "function (open:0)"=enum16{"open", "write", "close"}."close") -> ("error out"=w226:errorcluster)  [unwired: 4 in]
                                n188 = call "HandleError.vi"("error in (no error)"=w226) -> ()
                              }
                            }
                          }
                          frame #1 {
                            n189 = local read "Image Settings"() -> (w231:T2)
                            n190 = call "NextLine.vi"("Image Settings"=w231) -> ("Continue Scan"=w228:bool)
                            n191 = case shown="True" w228 {
                              tunnel: w229 -> [w232 _]
                              frame #0 {
                                n192 = stacked-sequence {
                                tunnel: w232 -> [w233 _ _ _]
                                frame #0 {
                                n193 = call "ScannedImage.vi"("Get/Set"=TRUE, "Scanned Image (input)"=w233) -> ()  [unwired: 1 out]
                                }
                                frame #1 {
                                n194 = local read "Display Settings"() -> (w235:T1)
                                n195 = call "UpdateFullImage.vi"("Display Settings"=w235) -> ()
                                }
                                frame #2 {
                                n196 = property on="Current Position (µm)" class="Cluster (strict)"() -> ("Value"=w237:cluster{"x":dbl, "y":dbl, "z":dbl})  [unwired: 2 in, 2 out]
                                n197 = call "SetPosition.vi"("Current Position (µm)"=w237) -> ("error out"=w236:errorcluster)
                                n198 = call "HandleError.vi"("error in (no error)"=w236) -> ()
                                }
                                frame #3 {
                                w238 = FALSE ("Laser 1")
                                n199 = call "AOTFSetPosition.vi"() -> ()  [unwired: 2 in]
                                n200 = property on="Laser 4" class="Boolesch (strikt)"("Value"=w238) -> ()  [unwired: 2 in, 2 out]
                                n201 = property on="Laser 1" class="Boolean (strict)"("Value"=w238) -> ()  [unwired: 2 in, 2 out]
                                n202 = property on="Laser 2" class="Boolean (strict)"("Value"=w238) -> ()  [unwired: 2 in, 2 out]
                                n203 = property on="Laser 3" class="Boolean (strict)"("Value"=w238) -> ()  [unwired: 2 in, 2 out]
                                }
                                }
                              }
                              frame #1 {
                                # "show position at end of line"
                                n204 = case shown="True" "show position (PI digital)" {
                                frame #0 {
                                }
                                frame #1 {
                                n205 = call "POS?.vi"("System no."=1, "All axes?"=TRUE) -> ("Position"=→"Position":dbl[])  [unwired: 16 in, 1 out]
                                }
                                }
                              }
                            }
                            n206 = call "UpdateFrontPanel.vi"("operation"=enum16{"set references", "update"}."update", "Scan"=w228) -> ()  [unwired: 8 in]
                            n207 = property on="Scan" class="Boolean (strict)"("Value"=w228) -> ()  [unwired: 2 in, 2 out]
                          }
                        }
                      }
                    }
                  }
                }
              }
            }
          }
          event #1 {
            n208 = event-data() -> ()  [unwired: 1 in, 1 out]
            n209 = Unbundle By Name("Current Position (µm)") -> ("x"=w244:dbl)
            n210 = Unbundle By Name("Position Increment (µm)") -> ("x"=w248:dbl)
            n211 = Subtract(x=w244, y=w248) -> (x-y=w245:dbl)
            n212 = Bundle By Name(cluster="Current Position (µm)", "x"=w245) -> (w243:cluster{"x":dbl, "y":dbl, "z":dbl})
            n213 = local read "Scan"() -> (w249:bool)
            n214 = case shown="True" w249 {
              tunnel: w243 -> [w251 w256]
              frame #0 {
                n215 = call "SetPosition.vi"("Current Position (µm)"=w251) -> ("error out"=w250:errorcluster)
                n216 = call "HandleError.vi"("error in (no error)"=w250) -> ()
              }
              frame #1 {
                n217 = Cluster To Array(cluster=w256) -> (array=w255:dbl[])
                n218 = local read "Image Settings"() -> (w259:T2)
                n219 = Unbundle By Name(w259) -> ("1st Axis"=w258:u16, "2nd Axis"=w257:u16)
                n220 = call "GetThirdAxis.vi"("1st Axis"=w257, "2nd Axis"=w258) -> ("3rd Axis"=w254:i32)  [unwired: 2 in]
                n221 = Index Array(array=w255, index=w254) -> (element=w253:dbl)
                n222 = call "SetAxisPos.vi"("Position"=w253, "Axis"=w254) -> ("error out"=w252:errorcluster)
                n223 = call "HandleError.vi"("error in (no error)"=w252) -> ()
              }
            }
            n224 = local write "Current Position (µm)"(w243) -> ()
          }
          event #2 {
            n225 = event-data() -> ()  [unwired: 1 in, 1 out]
            n226 = local read "Position Increment (µm)"() -> (w263:cluster{"x":dbl, "y":dbl, "z":dbl})
            n227 = local read "Current Position (µm)"() -> (w264:cluster{"x":dbl, "y":dbl, "z":dbl})
            n228 = Unbundle By Name(w264) -> ("x"=w265:dbl)
            n229 = Unbundle By Name(w263) -> ("x"=w262:dbl)
            n230 = Add(x=w265, y=w262) -> (x+y=w266:dbl)
            n231 = local read "Scan"() -> (w261:bool)
            n232 = Bundle By Name(cluster=w264, "x"=w266) -> (w260:cluster{"x":dbl, "y":dbl, "z":dbl})
            n233 = local write "Current Position (µm)"(w260) -> ()
            n234 = case shown="False" w261 {
              tunnel: w260 -> [w268 w271]
              frame #0 {
                n235 = call "SetPosition.vi"("Current Position (µm)"=w268) -> ("error out"=w267:errorcluster)
                n236 = call "HandleError.vi"("error in (no error)"=w267) -> ()
              }
              frame #1 {
                n237 = Cluster To Array(cluster=w271) -> (array=w273:dbl[])
                n238 = local read "Image Settings"() -> (w276:T2)
                n239 = Unbundle By Name(w276) -> ("1st Axis"=w275:u16, "2nd Axis"=w274:u16)
                n240 = call "GetThirdAxis.vi"("1st Axis"=w274, "2nd Axis"=w275) -> ("3rd Axis"=w272:i32)  [unwired: 2 in]
                n241 = Index Array(array=w273, index=w272) -> (element=w270:dbl)
                n242 = call "SetAxisPos.vi"("Position"=w270, "Axis"=w272) -> ("error out"=w269:errorcluster)
                n243 = call "HandleError.vi"("error in (no error)"=w269) -> ()
              }
            }
          }
          event #3 {
            n244 = event-data() -> ()  [unwired: 1 in, 1 out]
            n245 = local read "Position Increment (µm)"() -> (w282:cluster{"x":dbl, "y":dbl, "z":dbl})
            n246 = local read "Current Position (µm)"() -> (w279:cluster{"x":dbl, "y":dbl, "z":dbl})
            n247 = Unbundle By Name(w279) -> ("y"=w281:dbl)
            n248 = Unbundle By Name(w282) -> ("y"=w280:dbl)
            n249 = Add(x=w281, y=w280) -> (x+y=w283:dbl)
            n250 = local read "Scan"() -> (w278:bool)
            n251 = Bundle By Name(cluster=w279, "y"=w283) -> (w277:cluster{"x":dbl, "y":dbl, "z":dbl})
            n252 = local write "Current Position (µm)"(w277) -> ()
            n253 = case shown="False" w278 {
              tunnel: w277 -> [w285 w288]
              frame #0 {
                n254 = call "SetPosition.vi"("Current Position (µm)"=w285) -> ("error out"=w284:errorcluster)
                n255 = call "HandleError.vi"("error in (no error)"=w284) -> ()
              }
              frame #1 {
                n256 = Cluster To Array(cluster=w288) -> (array=w290:dbl[])
                n257 = local read "Image Settings"() -> (w293:T2)
                n258 = Unbundle By Name(w293) -> ("1st Axis"=w292:u16, "2nd Axis"=w291:u16)
                n259 = call "GetThirdAxis.vi"("1st Axis"=w291, "2nd Axis"=w292) -> ("3rd Axis"=w289:i32)  [unwired: 2 in]
                n260 = Index Array(array=w290, index=w289) -> (element=w287:dbl)
                n261 = call "SetAxisPos.vi"("Position"=w287, "Axis"=w289) -> ("error out"=w286:errorcluster)
                n262 = call "HandleError.vi"("error in (no error)"=w286) -> ()
              }
            }
          }
          event #4 {
            n263 = event-data() -> ()  [unwired: 1 in, 1 out]
            n264 = local read "Position Increment (µm)"() -> (w298:cluster{"x":dbl, "y":dbl, "z":dbl})
            n265 = local read "Current Position (µm)"() -> (w299:cluster{"x":dbl, "y":dbl, "z":dbl})
            n266 = Unbundle By Name(w299) -> ("y"=w296:dbl)
            n267 = Unbundle By Name(w298) -> ("y"=w297:dbl)
            n268 = Subtract(x=w296, y=w297) -> (x-y=w300:dbl)
            n269 = Bundle By Name(cluster=w299, "y"=w300) -> (w294:cluster{"x":dbl, "y":dbl, "z":dbl})
            n270 = local read "Scan"() -> (w295:bool)
            n271 = local write "Current Position (µm)"(w294) -> ()
            n272 = case shown="False" w295 {
              tunnel: w294 -> [w302 w305]
              frame #0 {
                n273 = call "SetPosition.vi"("Current Position (µm)"=w302) -> ("error out"=w301:errorcluster)
                n274 = call "HandleError.vi"("error in (no error)"=w301) -> ()
              }
              frame #1 {
                n275 = Cluster To Array(cluster=w305) -> (array=w307:dbl[])
                n276 = local read "Image Settings"() -> (w310:T2)
                n277 = Unbundle By Name(w310) -> ("1st Axis"=w309:u16, "2nd Axis"=w308:u16)
                n278 = call "GetThirdAxis.vi"("1st Axis"=w308, "2nd Axis"=w309) -> ("3rd Axis"=w306:i32)  [unwired: 2 in]
                n279 = Index Array(array=w307, index=w306) -> (element=w304:dbl)
                n280 = call "SetAxisPos.vi"("Position"=w304, "Axis"=w306) -> ("error out"=w303:errorcluster)
                n281 = call "HandleError.vi"("error in (no error)"=w303) -> ()
              }
            }
          }
          event #5 {
            n282 = event-data() -> ()  [unwired: 1 in, 1 out]
            n283 = local read "Position Increment (µm)"() -> (w316:cluster{"x":dbl, "y":dbl, "z":dbl})
            n284 = local read "Current Position (µm)"() -> (w313:cluster{"x":dbl, "y":dbl, "z":dbl})
            n285 = Unbundle By Name(w316) -> ("z"=w314:dbl)
            n286 = Unbundle By Name(w313) -> ("z"=w315:dbl)
            n287 = Add(x=w315, y=w314) -> (x+y=w317:dbl)
            n288 = Bundle By Name(cluster=w313, "z"=w317) -> (w311:cluster{"x":dbl, "y":dbl, "z":dbl})
            n289 = local write "Current Position (µm)"(w311) -> ()
            n290 = local read "Scan"() -> (w312:bool)
            n291 = case shown="False" w312 {
              tunnel: w311 -> [w319 w322]
              frame #0 {
                n292 = call "SetPosition.vi"("Current Position (µm)"=w319) -> ("error out"=w318:errorcluster)
                n293 = call "HandleError.vi"("error in (no error)"=w318) -> ()
              }
              frame #1 {
                n294 = Cluster To Array(cluster=w322) -> (array=w324:dbl[])
                n295 = local read "Image Settings"() -> (w327:T2)
                n296 = Unbundle By Name(w327) -> ("1st Axis"=w326:u16, "2nd Axis"=w325:u16)
                n297 = call "GetThirdAxis.vi"("1st Axis"=w325, "2nd Axis"=w326) -> ("3rd Axis"=w323:i32)  [unwired: 2 in]
                n298 = Index Array(array=w324, index=w323) -> (element=w321:dbl)
                n299 = call "SetAxisPos.vi"("Position"=w321, "Axis"=w323) -> ("error out"=w320:errorcluster)
                n300 = call "HandleError.vi"("error in (no error)"=w320) -> ()
              }
            }
          }
          event #6 {
            n301 = event-data() -> ()  [unwired: 1 in, 1 out]
            n302 = local read "Position Increment (µm)"() -> (w334:cluster{"x":dbl, "y":dbl, "z":dbl})
            n303 = local read "Current Position (µm)"() -> (w330:cluster{"x":dbl, "y":dbl, "z":dbl})
            n304 = Unbundle By Name(w330) -> ("z"=w333:dbl)
            n305 = Unbundle By Name(w334) -> ("z"=w332:dbl)
            n306 = Subtract(x=w333, y=w332) -> (x-y=w331:dbl)
            n307 = Bundle By Name(cluster=w330, "z"=w331) -> (w328:cluster{"x":dbl, "y":dbl, "z":dbl})
            n308 = local read "Scan"() -> (w329:bool)
            n309 = local write "Current Position (µm)"(w328) -> ()
            n310 = case shown="False" w329 {
              tunnel: w328 -> [w336 w339]
              frame #0 {
                n311 = call "SetPosition.vi"("Current Position (µm)"=w336) -> ("error out"=w335:errorcluster)
                n312 = call "HandleError.vi"("error in (no error)"=w335) -> ()
              }
              frame #1 {
                n313 = Cluster To Array(cluster=w339) -> (array=w341:dbl[])
                n314 = local read "Image Settings"() -> (w344:T2)
                n315 = Unbundle By Name(w344) -> ("1st Axis"=w343:u16, "2nd Axis"=w342:u16)
                n316 = call "GetThirdAxis.vi"("1st Axis"=w342, "2nd Axis"=w343) -> ("3rd Axis"=w340:i32)  [unwired: 2 in]
                n317 = Index Array(array=w341, index=w340) -> (element=w338:dbl)
                n318 = call "SetAxisPos.vi"("Position"=w338, "Axis"=w340) -> ("error out"=w337:errorcluster)
                n319 = call "HandleError.vi"("error in (no error)"=w337) -> ()
              }
            }
          }
          event #7 {
            n320 = event-data() -> ()  [unwired: 1 in, 1 out]
            n321 = local read "Current Position (µm)"() -> (w345:cluster{"x":dbl, "y":dbl, "z":dbl})
            n322 = Unbundle By Name(w345) -> ("x"=w351:dbl, "y"=w350:dbl, "z"=w348:dbl)
            n323 = Bundle("x"=w351, "y"=w350, "z"=w348) -> (w349:cluster{"x":dbl, "y":dbl, "z":dbl})  [unwired: 1 in]
            n324 = case shown="True" "Keep Start Position" {
              tunnel: w349 -> [w352 w362]
              tunnel: "Keep Image Size" -> [w353 w363]
              frame #0 {
                n325 = property on="Start Position (µm)" class="Clust (strict)"("Value"=w352) -> ()  [unwired: 2 in, 2 out]
                n326 = case shown="False" w353 {
                  tunnel: w352 -> [w354 w357]
                  frame #0 {
                    n327 = property on="Image Size (µm)" class="Clust (strict)"() -> ("Value"=w355:cluster{"x":dbl, "y":dbl, "z":dbl})  [unwired: 2 in, 2 out]
                    n328 = Add(x=w355, y=w354) -> (x+y=w356:cluster{"x":dbl, "y":dbl, "z":dbl})
                    n329 = property on="End Position (µm)" class="Clust (strict)"("Value"=w356) -> ()  [unwired: 2 in, 2 out]
                  }
                  frame #1 {
                    n330 = stacked-sequence {
                      tunnel: w357 -> [w358 _]
                      frame #0 {
                        n331 = property on="End Position (µm)" class="Clust (strict)"() -> ("Value"=w360:cluster{"x":dbl, "y":dbl, "z":dbl})  [unwired: 2 in, 2 out]
                        n332 = Subtract(x=w360, y=w358) -> (x-y=w359:cluster{"x":dbl, "y":dbl, "z":dbl})
                        n333 = property on="Image Size (µm)" class="Clust (strict)"("Value"=w359) -> ()  [unwired: 2 in, 2 out]
                      }
                      frame #1 {
                        n334 = call "UpdateImageInfo.vi"("operation"=enum16{"set references", "update"}."update") -> ()  [unwired: 3 in]
                      }
                    }
                  }
                }
              }
              frame #1 {
                n335 = property on="End Position (µm)" class="Clust (strict)"("Value"=w362) -> ()  [unwired: 2 in, 2 out]
                n336 = case shown="False" w363 {
                  tunnel: w362 -> [w364 w367]
                  frame #0 {
                    n337 = property on="Image Size (µm)" class="Clust (strict)"() -> ("Value"=w366:cluster{"x":dbl, "y":dbl, "z":dbl})  [unwired: 2 in, 2 out]
                    n338 = Subtract(x=w364, y=w366) -> (x-y=w365:cluster{"x":dbl, "y":dbl, "z":dbl})
                    n339 = property on="Start Position (µm)" class="Clust (strict)"("Value"=w365) -> ()  [unwired: 2 in, 2 out]
                  }
                  frame #1 {
                    n340 = stacked-sequence {
                      tunnel: w367 -> [w368 _]
                      frame #0 {
                        n341 = property on="Start Position (µm)" class="Clust (strict)"() -> ("Value"=w370:cluster{"x":dbl, "y":dbl, "z":dbl})  [unwired: 2 in, 2 out]
                        n342 = Subtract(x=w368, y=w370) -> (x-y=w369:cluster{"x":dbl, "y":dbl, "z":dbl})
                        n343 = property on="Image Size (µm)" class="Clust (strict)"("Value"=w369) -> ()  [unwired: 2 in, 2 out]
                      }
                      frame #1 {
                        n344 = call "UpdateImageInfo.vi"("operation"=enum16{"set references", "update"}."update") -> ()  [unwired: 3 in]
                      }
                    }
                  }
                }
              }
            }
          }
          event #8 {
            n345 = event-data() -> ("NewVal"=w373:bool)  [unwired: 1 in]
            n346 = control-ref of="y"() -> (w374:refnum<vi>)
            n347 = case shown="True" w373 {
              frame #0 {
              }
              frame #1 {
                n348 = stacked-sequence {
                  frame #0 {
                    n349 = property on="Image Resolution (nm/pixel)" class="Clust (strict)"() -> ("Value"=w378:cluster{"x":dbl, "y":dbl, "z":dbl})  [unwired: 2 in, 2 out]
                    n350 = Unbundle(w378) -> ("x"=w377:dbl, "z"=w375:dbl)  [unwired: 1 out]
                    n351 = Bundle("x"=w377, "x"=w377, "z"=w375) -> (w376:cluster{"x":dbl, "x":dbl, "z":dbl})  [unwired: 1 in]
                    n352 = property on="Image Resolution (nm/pixel)" class="Clust (strict)"("Value"=w376) -> ()  [unwired: 2 in, 2 out]
                  }
                  frame #1 {
                    n353 = call "UpdateImageInfo.vi"() -> ()  [unwired: 4 in]
                  }
                }
              }
            }
            n354 = Not(x=w373) -> (.not. x?=w372:bool)
            n355 = call "EnableControl.vi"("Enable"=w372, "Reference"=w374) -> ()
          }
          event #9 {
            n356 = event-data() -> ("NewVal"=w380:cluster{"x":dbl, "y":dbl, "z":dbl})  [unwired: 1 in]
            n357 = local read "Keep Image Size"() -> (w379:bool)
            n358 = case shown="False" w379 {
              tunnel: w380 -> [w383 w384]
              frame #0 {
                n359 = property on="Image Size (µm)" class="Clust (strict)"() -> ("Value"=w381:cluster{"x":dbl, "y":dbl, "z":dbl})  [unwired: 2 in, 2 out]
                n360 = Add(x=w381, y=w383) -> (x+y=w382:cluster{"x":dbl, "y":dbl, "z":dbl})
                n361 = property on="End Position (µm)" class="Clust (strict)"("Value"=w382) -> ()  [unwired: 2 in, 2 out]
              }
              frame #1 {
                n362 = stacked-sequence {
                  tunnel: w384 -> [w387 _]
                  frame #0 {
                    n363 = property on="End Position (µm)" class="Cluster (strict)"() -> ("Value"=w386:cluster{"x":dbl, "y":dbl, "z":dbl})  [unwired: 2 in, 2 out]
                    n364 = Subtract(x=w386, y=w387) -> (x-y=w385:cluster{"x":dbl, "y":dbl, "z":dbl})
                    n365 = property on="Image Size (µm)" class="Cluster (strict)"("Value"=w385) -> ()  [unwired: 2 in, 2 out]
                  }
                  frame #1 {
                    n366 = call "UpdateImageInfo.vi"() -> ()  [unwired: 4 in]
                  }
                }
              }
            }
          }
          event #10 {
            n367 = event-data() -> ("NewVal"=w389:cluster{"x":dbl, "y":dbl, "z":dbl})  [unwired: 1 in]
            n368 = local read "Keep Image Size"() -> (w388:bool)
            n369 = case shown="False" w388 {
              tunnel: w389 -> [w391 w393]
              frame #0 {
                n370 = property on="Image Size (µm)" class="Clust (strict)"() -> ("Value"=w392:cluster{"x":dbl, "y":dbl, "z":dbl})  [unwired: 2 in, 2 out]
                n371 = Subtract(x=w391, y=w392) -> (x-y=w390:cluster{"x":dbl, "y":dbl, "z":dbl})
                n372 = property on="Start Position (µm)" class="Clust (strict)"("Value"=w390) -> ()  [unwired: 2 in, 2 out]
              }
              frame #1 {
                n373 = stacked-sequence {
                  tunnel: w393 -> [w396 _]
                  frame #0 {
                    n374 = property on="Start Position (µm)" class="Clust (strict)"() -> ("Value"=w395:cluster{"x":dbl, "y":dbl, "z":dbl})  [unwired: 2 in, 2 out]
                    n375 = Subtract(x=w396, y=w395) -> (x-y=w394:cluster{"x":dbl, "y":dbl, "z":dbl})
                    n376 = property on="Image Size (µm)" class="Clust (strict)"("Value"=w394) -> ()  [unwired: 2 in, 2 out]
                  }
                  frame #1 {
                    n377 = call "UpdateImageInfo.vi"() -> ()  [unwired: 4 in]
                  }
                }
              }
            }
          }
          event #11 {
            n378 = event-data() -> ("NewVal"=w397:cluster{"x":dbl, "y":dbl, "z":dbl})  [unwired: 1 in]
            n379 = stacked-sequence {
              tunnel: w397 -> [w399 _]
              frame #0 {
                n380 = local read "Keep Start Position"() -> (w398:bool)
                n381 = case shown="False" w398 {
                  tunnel: w399 -> [w400 w403]
                  frame #0 {
                    n382 = property on="Start Position (µm)" class="Clust (strict)"() -> ("Value"=w402:cluster{"x":dbl, "y":dbl, "z":dbl})  [unwired: 2 in, 2 out]
                    n383 = Add(x=w400, y=w402) -> (x+y=w401:cluster{"x":dbl, "y":dbl, "z":dbl})
                    n384 = property on="End Position (µm)" class="Clust (strict)"("Value"=w401) -> ()  [unwired: 2 in, 2 out]
                  }
                  frame #1 {
                    n385 = property on="End Position (µm)" class="Clust (strict)"() -> ("Value"=w404:cluster{"x":dbl, "y":dbl, "z":dbl})  [unwired: 2 in, 2 out]
                    n386 = Subtract(x=w404, y=w403) -> (x-y=w405:cluster{"x":dbl, "y":dbl, "z":dbl})
                    n387 = property on="Start Position (µm)" class="Clust (strict)"("Value"=w405) -> ()  [unwired: 2 in, 2 out]
                  }
                }
              }
              frame #1 {
                n388 = call "UpdateImageInfo.vi"("operation"=enum16{"set references", "update"}."update") -> ()  [unwired: 3 in]
              }
            }
          }
          event #12 {
            n389 = event-data() -> ()  [unwired: 1 in, 5 out]
            n390 = call "UpdateImageInfo.vi"() -> ()  [unwired: 4 in]
            n391 = local read "Image Settings"() -> (w415:T2)
            n392 = Unbundle By Name(w415) -> ("Time Resolution\n(ms/pixel)"=w414:dbl)
            n393 = Reciprocal(x=w414) -> (1/x=w413:dbl)
            n394 = Select(t=w413, s="x-scale: Time?", f=1.0) -> (s? t:f=w412:dbl)
            n395 = Select(t="Time [ms]", s="x-scale: Time?", f="Pixel") -> (s? t:f=w409:string)
            n396 = property on="MCS Trace" class="WaveformChart (strict)"("X Scale.Offset and Multiplier:Multiplier"=w412, "X Scale.Name Label.Text"=w409) -> ()  [unwired: 2 in, 2 out]
          }
          event #13 {
            n397 = event-data() -> ("NewVal"=w420:bool)  [unwired: 1 in, 4 out]
            n398 = property on="Show Image" class="Boolean (strict)"() -> ("Value"=w416:bool)  [unwired: 2 in, 2 out]
            n399 = call "DAQLinescanVisualization.vi"() -> ("Visualization (output)"=w419:T6)  [unwired: 2 in]
            n400 = And(x=w420, y=w416) -> (x .and. y?=w417:bool)
            n401 = Unbundle By Name(w419) -> ("Retrace Window #"=w418:u32)
            n402 = call "IMAQ WindShow"("Bring To Front? (N)"=w417, "Hide/Show (Show)"=w417, "Window Number (0...15)"=w418) -> ()  [unwired: 3 in, 3 out]
          }
          event #14 {
            n403 = event-data() -> ("Time"=w421:u32, "NewVal"=w423:bool)  [unwired: 1 in, 3 out]
            n404 = call "DAQLinescanVisualization.vi"() -> ("Visualization (output)"=w429:T6)  [unwired: 2 in]
            n405 = property on="Retrace" class="Boolean (strict)"() -> ("Value"=w425:bool)  [unwired: 2 in, 2 out]
            n406 = Unbundle By Name(w429) -> ("Trace Window #"=w428:u32, "Retrace Window #"=w427:u32)
            n407 = control-ref of="Plane"() -> (w424:refnum<vi>)
            n408 = And(x=w425, y=w423) -> (x .and. y?=w426:bool)
            n409 = Multiply(x=w421, y=w428) -> (x*y=w422:u32)
            n410 = call "IMAQ WindToolsShow"("Hide/Show (Show)"=w423) -> ()  [unwired: 4 in, 2 out]
            n411 = call "IMAQ WindShow"("Bring To Front? (N)"=w423, "Hide/Show (Show)"=w423, "Window Number (0...15)"=w422) -> ()  [unwired: 3 in, 3 out]
            n412 = call "IMAQ WindShow"("Bring To Front? (N)"=w426, "Hide/Show (Show)"=w426, "Window Number (0...15)"=w427) -> ()  [unwired: 3 in, 3 out]
            n413 = call "EnableControl.vi"("Enable"=w423, "Reference"=w424) -> ()
          }
          event #15 {
            n414 = event-data() -> ()  [unwired: 1 in, 5 out]
            n415 = control-ref of="Load Image"() -> (w430:refnum<vi>)
            n416 = control-ref of="Scan"() -> ()  [unwired: 1 out]
            n417 = call "BuildHdrFilePath.vi"("Destination:"="Destination:") -> ("error in (no error)"=w432:errorcluster, "configuration file path"=w433:path)  [unwired: 1 in]
            n418 = call "UpdateSomeButtons.vi"("Load"=w430, "Destination:"=w433, "error in (no error)"=w432, "Store Data"="Store Data") -> ("error"=w431:errorcluster)  [unwired: 1 in]
            n419 = call "HandleError.vi"("error in (no error)"=w431) -> ()
          }
          event #16 {
            n420 = event-data() -> ()  [unwired: 1 in, 5 out]
            n421 = Select(t=u8 2 ("Y Scale.Scale Fit"), s="Autoscale y-axis", f=u8 0 ("Y Scale.Scale Fit")) -> (s? t:f=w438:u8)
            n422 = property on="MCS Trace" class="WaveformChart (strict)"("Y Scale.Scale Fit"=w438) -> ()  [unwired: 2 in, 2 out]
          }
          event #17 {
            n423 = event-data() -> ()  [unwired: 1 in, 5 out]
            n424 = property on="Scan" class="Boolean (strict)"() -> ("Value"=w440:bool)  [unwired: 2 in, 2 out]
            n425 = case shown="False" w440 {
              frame #0 {
                n426 = call "UpdateFullImage.vi"("Display Settings"="Display Settings") -> ()
              }
              frame #1 {
              }
            }
          }
          event #18 {
            n427 = event-data() -> ()  [unwired: 1 in, 1 out]
            n428 = case shown="True" "EOM Setup" {
              frame #0 {
              }
              frame #1 {
                n429 = stacked-sequence {
                  frame #0 {
                    n430 = property class="VI"() -> ("VI Name"=w444:string)  [unwired: 2 in, 2 out]
                    n431 = call "CallersName.vi"("Get/Set"=TRUE ("s"), "Callers Name"=w444) -> ()  [unwired: 1 out]
                  }
                  frame #1 {
                    n432 = call "SetupEOM.vi"() -> ()  [unwired: 1 in]
                  }
                }
              }
            }
          }
          event #19 {
            n433 = event-data() -> ("NewVal"=w446:u16)  [unwired: 1 in, 4 out]
            n434 = flat-sequence {
              tunnel: w446 -> [w451]
              tunnel: [w451] -> w445
              tunnel: w445 -> [w455]
              frame #0 {
                n435 = property on="AOTF" class="Ring (strict)"() -> ("Value"=w448:u16)  [unwired: 2 in, 2 out]
                n436 = Not Equal To 0?(x=w451) -> (x != 0?=w452:bool)
                n437 = Equal?(x=u8 7, y=w448) -> (x = y?=w447:bool)
                n438 = And(x=w452, y=w447) -> (x .and. y?=w450:bool)
                n439 = case shown="True" w450 {
                  frame #0 {
                  }
                  frame #1 {
                    w454 = u16 3 items=["None", "Laser 1", "Laser 2", "Laser 1 + 2", "Laser 3", "Laser 1 + 3", "Laser 2 + 3", "Laser 1+2+3"] ("AOTF")
                    n440 = control-ref of="AOTF"() -> (w453:refnum<vi>)
                    n441 = call "Display Message to User"() -> ()  [unwired: 10 in, 2 out]
                    n442 = property on="Property Node" class="Ring (strict)"(reference=w453, "Value"=w454) -> ()  [unwired: 1 in, 2 out]
                  }
                }
              }
              frame #1 {
                n443 = case shown="1, Default" w455 {
                  frame #0 {
                  }
                  frame #1 {
                    n444 = call "EOMSetPosition.vi"("value"=sgl 0.0) -> ()
                  }
                }
              }
            }
          }
          event #20 {
            n445 = event-data() -> ()  [unwired: 1 in, 1 out]
            n446 = case shown="True" "Stage Setup" {
              frame #0 {
              }
              frame #1 {
                n447 = stacked-sequence {
                  frame #0 {
                    n448 = call "StageType.vi"() -> ()  [unwired: 3 in, 3 out]
                  }
                  frame #1 {
                    n449 = call "SetupStage.vi"() -> ()  [unwired: 1 in]
                  }
                  frame #2 {
                    n450 = call "StageInit.vi"() -> ("error out"=w458:errorcluster)  [unwired: 1 in]
                    n451 = case shown="No Error" w458 {
                      selector: w458 -> [_ w462]
                      tunnel: [w460 w462] -> w459
                      frame #0 {
                        n452 = property on="Current Position (µm)" class="Clust (strict)"() -> ("Value"=w461:cluster{"x":dbl, "y":dbl, "z":dbl})  [unwired: 2 in, 2 out]
                        n453 = call "SetPosition.vi"("Current Position (µm)"=w461) -> ("error out"=w460:errorcluster)
                      }
                      frame #1 {
                      }
                    }
                    n454 = call "HandleError.vi"("error in (no error)"=w459) -> ()
                  }
                }
              }
            }
          }
          event #21 {
            n455 = event-data() -> ()  [unwired: 1 in, 6 out]
            n456 = case shown="True" "AOTF Setup" {
              frame #0 {
              }
              frame #1 {
                n457 = stacked-sequence {
                  frame #0 {
                    n458 = property class="VI"() -> ("VI Name"=w465:string)  [unwired: 2 in, 2 out]
                    n459 = call "CallersName.vi"("Get/Set"=TRUE ("s"), "Callers Name"=w465) -> ()  [unwired: 1 out]
                  }
                  frame #1 {
                    n460 = call "SetupAOTF.vi"() -> ()  [unwired: 1 in]
                  }
                }
              }
            }
          }
          event #22 {
            n461 = event-data() -> ("NewVal"=w466:u16)  [unwired: 1 in, 5 out]
            n462 = flat-sequence {
              tunnel: w466 -> [w467]
              frame #0 {
                n463 = Equal?(x=u8 7, y=w467) -> (x = y?=w472:bool)
                n464 = property on="EOM" class="Ring (strict)"() -> ("Value"=w468:u16)  [unwired: 2 in, 2 out]
                n465 = Not Equal To 0?(x=w468) -> (x != 0?=w469:bool)
                n466 = And(x=w469, y=w472) -> (x .and. y?=w470:bool)
                n467 = case shown="True" w470 {
                  frame #0 {
                  }
                  frame #1 {
                    w473 = u16 3 items=["None", "Laser 1", "Laser 2", "Laser 1 + 2", "Laser 3", "Laser 1 + 3", "Laser 2 + 3", "Laser 1+2+3"] ("AOTF")
                    n468 = call "Display Message to User2"() -> ()  [unwired: 10 in, 2 out]
                    n469 = property on="AOTF" class="Ring (strict)"("Value"=w473) -> ()  [unwired: 2 in, 2 out]
                  }
                }
              }
              frame #1 {
                n470 = call "AOTFSetPosition.vi"() -> ()  [unwired: 2 in]
              }
            }
          }
          event #23 {
            n471 = event-data() -> ("ItemTag"=w474:string)  [unwired: 1 in, 5 out]
            n472 = case shown="\"\", Default" w474 {
              frame #0 {
              }
              frame #1 {
                n473 = call "Splashscreen.vi"("Mode"=enum16{"splash", "dialog"}."dialog") -> ()  [unwired: 1 in]
              }
            }
          }
          event #24 {
            n474 = event-data() -> ()  [unwired: 1 in, 1 out]
            n475 = case shown="True" "SPC Setup" {
              frame #0 {
              }
              frame #1 {
                n476 = stacked-sequence {
                  frame #0 {
                    w477 = u16 1 items=["standalone", "dialog"] ("mode")
                    n477 = call "DAQFIFO_HH.vi"("mode"=w477) -> ()
                  }
                  frame #1 {
                    n478 = call "FIFOSettings.vi"() -> ("FIFO Settings(out)"=w478:T5)  [unwired: 2 in]
                    n479 = call "SPCSetParameters_HH.vi"("FIFO Settings"=w478) -> ("error (out)"=w479:errorcluster)  [unwired: 2 in]
                    n480 = call "HandleError.vi"("error in (no error)"=w479) -> ()
                  }
                  frame #2 {
                    n481 = property class="VI"() -> (error out=w480:errorcluster, "Front Panel"=w481:refnum<vi>)  [unwired: 2 in, 1 out]
                    n482 = call "UpdateDAQLinescanStatus.vi"("error in (no error)"=w480, "Panel"=w481) -> ()
                  }
                }
              }
            }
          }
          event #25 {
            n483 = event-data() -> ()  [unwired: 1 in, 1 out]
            n484 = stacked-sequence {
              frame #0 {
                n485 = case shown="True" "Save & Exit" {
                  frame #0 {
                  }
                  frame #1 {
                    n486 = call "WriteAnalogSettings.vi"() -> ("error out"=w487:errorcluster)  [unwired: 1 in]
                    n487 = call "WriteStageSettings.vi"("error in (no error)"=w487) -> ("error out"=w486:errorcluster)
                    n488 = call "WriteEOMSettings.vi"("error in (no error)"=w486) -> ("error out"=w485:errorcluster)
                    n489 = call "WriteAOTFSettings.vi"("error in (no error)"=w485) -> ("error out"=w484:errorcluster)
                    n490 = call "HandleError.vi"("error in (no error)"=w484) -> ()
                  }
                }
              }
              frame #1 {
                n491 = property class="VI"("Front Panel Window:Open"=TRUE) -> ()  [unwired: 2 in, 2 out]
              }
            }
          }
          event #26 {
            n492 = event-data() -> ("NewVal"=w489:bool)  [unwired: 1 in]
            n493 = call "UpdateFrontPanel.vi"("operation"=enum16{"set references", "update"}."update", "Scan"=w489) -> ()  [unwired: 8 in]
            n494 = case shown="True" w489 {
              frame #0 {
                n495 = stacked-sequence {
                  frame #0 {
                    n496 = call "OperateOnAnalogOutput.vi"("operation"=enum16{"start", "state", "abort"}."abort") -> ("error out"=w491:errorcluster)  [unwired: 1 in, 1 out]
                    n497 = call "HandleError.vi"("error in (no error)"=w491) -> ()
                  }
                  frame #1 {
                    n498 = call "HaltStageOutput.vi"() -> ("Error out"=w493:errorcluster)  [unwired: 1 in]
                    n499 = call "HandleError.vi"("error in (no error)"=w493) -> ()
                  }
                  frame #2 {
                    n500 = call "FIFOStopDAQ.vi"() -> ("error out"=w494:errorcluster)
                    n501 = call "HandleError.vi"("error in (no error)"=w494) -> ()
                  }
                  frame #3 {
                    n502 = property on="Current Position (µm)" class="Cluster (strict)"() -> ("Value"=w496:cluster{"x":dbl, "y":dbl, "z":dbl})  [unwired: 2 in, 2 out]
                    n503 = call "SetPosition.vi"("Current Position (µm)"=w496) -> ("error out"=w495:errorcluster)
                    n504 = call "HandleError.vi"("error in (no error)"=w495) -> ()
                  }
                  frame #4 {
                    n505 = call "FIFOFileObject.vi"(".sm file format"=FALSE, "function (open:0)"=enum16{"open", "write", "close"}."close") -> ("error out"=w499:errorcluster)  [unwired: 4 in]
                    n506 = call "HandleError.vi"("error in (no error)"=w499) -> ()
                  }
                  frame #5 {
                    n507 = call "UpdateDAQLinescanImage.vi"("operation"=enum16{"initialize", "update", "read"}."read") -> ("LinescanSampling"=w502:T11)  [unwired: 3 in, 1 out]
                    n508 = call "ScannedImage.vi"("Get/Set"=TRUE, "Scanned Image (input)"=w502) -> ()  [unwired: 1 out]
                  }
                  frame #6 {
                    n509 = local read "Display Settings"() -> (w503:T1)
                    n510 = call "UpdateFullImage.vi"("Display Settings"=w503) -> ()
                  }
                  frame #7 {
                    n511 = call "AOTFSetPosition.vi"() -> ()  [unwired: 2 in]
                  }
                }
              }
              frame #1 {
                n512 = call <vilib>:"Initialize Mouse.vi"() -> ("device ID"=w508:refnum<k1>)  [unwired: 10 in, 1 out]
                n513 = call-poly <vilib>:"Acquire Input Data.vi"("device ID"=w508) -> ("device ID"=w506:refnum<k1>, "axis info"=w507:T12)  [unwired: 15 in, 2 out]
                n514 = Unbundle By Name(w507) -> ("Scrolling"=w505:i32)
                n515 = Bundle("device ID"=w506, "Scrolling"=w505) -> (→"mouse focus":cluster{"device ID":refnum<k1>, "Scrolling":i32})  [unwired: 1 in]
                n516 = call "InitializeAnalogOutput.vi"("AOTF"="AOTF", "% puls-duration"=100.0, "Image Settings"="Image Settings", "EOM"="EOM") -> ("Error out"=w513:errorcluster)
                n517 = case shown="No Error" w513 {
                  selector: w513 -> [w516 w542]
                  tunnel: "Image Settings" -> [w518 _]
                  tunnel: [w517 w542] -> w512
                  frame #0 {
                    w536 = u16 0 items=["initialize", "update"] ("operation")
                    n518 = Unbundle By Name(w518) -> ("1st Axis"=w528:u16, "2nd Axis"=w529:u16, "Image Size (pixel)"=w530:cluster{"x":u32, "y":u32, "z":u32})
                    n519 = control-ref of="MCS Trace"() -> (w533:refnum<vi>)
                    n520 = call "FIFOInitDAQ_HH.vi"() -> ()  [unwired: 1 in]
                    n521 = control-ref of="Image Settings"() -> (w534:refnum<vi>)
                    n522 = control-ref of="Display Settings"() -> (w535:refnum<vi>)
                    n523 = Cluster To Array(cluster=w530) -> (array=w527:u32[])
                    n524 = call "GetThirdAxis.vi"("1st Axis"=w529, "2nd Axis"=w528) -> ("3rd Axis"=w526:i32)  [unwired: 2 in]
                    n525 = call "UpdateDAQLinescanDisplay.vi"("MCS Trace"=w533, "operation"=enum16{"initialize", "update"}."initialize", "Display Settings"=w535, "Image Settings"=w534) -> ()  [unwired: 1 in]
                    n526 = Index Array(array=w527, index=w526) -> (element=w524:u32)
                    n527 = call "ImageParameters.vi"("Get/Set"=TRUE, "Image Parameters (input)"=w518) -> ()  [unwired: 1 out]
                    n528 = property on="Store Data" class="Boolean (strict)"() -> ("Value"=w519:bool)  [unwired: 2 in, 2 out]
                    n529 = call "UpdateDAQLinescanImage.vi"("Image Settings"=w534, "operation"=w536) -> ()  [unwired: 2 in, 2 out]
                    n530 = Not Equal To 0?(x=w524) -> (x != 0?=w525:bool)
                    n531 = Decrement(x=w524) -> (x-1=w520:u32)
                    n532 = case shown="False" w519 {
                      tunnel: w518 -> [_ w540]
                      tunnel: [w537 w539] -> w517
                      tunnel: w516 -> [w537 w538]
                      frame #0 {
                      }
                      frame #1 {
                        n533 = property on="Destination:" class="Path"() -> ("Value"=w541:path)  [unwired: 2 in, 2 out]
                        n534 = call "WriteLinescanHeader.vi"("error in"=w538, "Destination:"=w541, "Image Settings"=w540) -> ("error out"=w539:errorcluster)
                      }
                    }
                    n535 = Select(t=w520, s=w525, f=u32 0) -> (s? t:f=w521:u32)
                    n536 = property on="Plane" class="DigNum (strict)"() -> ("Data Entry Limits"=w522:T13)  [unwired: 2 in, 2 out]
                    n537 = Bundle By Name(cluster=w522, "Maximum"=w521) -> (w515:T13)
                    n538 = property on="Plane" class="DigNum (strict)"("Data Entry Limits"=w515) -> ()  [unwired: 2 in, 2 out]
                  }
                  frame #1 {
                  }
                }
                n539 = call "HandleError.vi"("error in (no error)"=w512) -> ()
              }
            }
          }
          event #27 {
            n540 = event-data() -> ()  [unwired: 1 in, 1 out]
            n541 = property on="show position (PI digital)" class="Bool (strict)"() -> ("Value"=w543:bool)  [unwired: 2 in, 2 out]
            n542 = case shown="False" w543 {
              frame #0 {
                n543 = property on="Numeric" class="DigNum (strict)"("Visible"=FALSE) -> ()  [unwired: 2 in, 2 out]
                n544 = property on="Position" class="Arr (strict)"("Visible"=FALSE) -> ()  [unwired: 2 in, 2 out]
              }
              frame #1 {
                n545 = call "POS?.vi"("System no."=1, "All axes?"=TRUE) -> ("Position"=w547:dbl[])  [unwired: 16 in, 1 out]
                n546 = property on="Numeric" class="DigNum (strict)"("Visible"=TRUE) -> ()  [unwired: 2 in, 2 out]
                n547 = property on="Position" class="Arr (strict)"("Visible"=TRUE) -> ()  [unwired: 2 in, 2 out]
                n548 = local write "Position"(w547) -> ()
              }
            }
          }
          event #28 {
            n549 = event-data() -> ()  [unwired: 1 in, 5 out]
            n550 = local read "Display Settings"() -> (w551:T1)
            n551 = stacked-sequence {
              tunnel: w551 -> [_ w558 w564]
              frame #0 {
              }
              frame #1 {
                w553 = 0 ("index (vol)")
                n552 = call "ScannedImage.vi"() -> ("Scanned Image (output)"=w557:T11)  [unwired: 2 in]
                n553 = Unbundle By Name(w558) -> ("Plane"=w556:u32, "Threshold.max"=w555:u32)
                n554 = Unbundle By Name(w557) -> ("Trace"=w554:u32[][][][])
                n555 = call "ExtractImagePlane.vi"("Router"=w555, "Plane"=w556, "Trace"=w554) -> ()  [unwired: 1 out]
                n556 = local read "Image Settings"() -> (w559:T2)
                n557 = Index Array(array=w554, index (dim 0)=w553, index (dim 1)=w553) -> (element=w552:u32[][])  [unwired: 2 in]
                n558 = call "PickAndDestroy.vi"("Image Settings"=w559, "Threshold"=w555, "Image"=w552) -> ()
              }
              frame #2 {
                n559 = call "FIFOSettings.vi"() -> ("FIFO Settings(out)"=w562:T5)  [unwired: 2 in]
                n560 = call "UpdateFullImage.vi"("Display Settings"=w564) -> ()
                n561 = call "SPCSetParameters_HH.vi"("FIFO Settings"=w562) -> ("error (out)"=w563:errorcluster)  [unwired: 2 in]
                n562 = property class="VI"() -> ("VI Name"=w561:string)  [unwired: 2 in, 2 out]
                n563 = call "HandleError.vi"("error in (no error)"=w563) -> ()
                n564 = call "CallersName.vi"("Get/Set"=TRUE ("s"), "Callers Name"=w561) -> ()  [unwired: 1 out]
              }
            }
          }
          event #29 {
            n565 = event-data() -> ()  [unwired: 1 in, 5 out]
          }
          event #30 {
            n566 = event-data() -> ()  [unwired: 1 in, 6 out]
            n567 = call "AnalogSettings.vi"() -> ("Analog Settings (output)"=w568:T14)  [unwired: 2 in]
            n568 = call "AOTFSettings.vi"() -> ("AOTF Setting (Output)"=w569:T15)  [unwired: 2 in]
            n569 = Unbundle By Name(w569) -> ("Laser 1 Output Channel"=w566:tag, "AOTF  1 Output Voltage"=w565:dbl)
            n570 = Unbundle By Name(w568) -> ("PCI 671x Device Number"=w567:u32)
            n571 = case shown="True" "Laser 1" {
              tunnel: w567 -> [w572 w575]
              tunnel: w566 -> [w571 w576]
              tunnel: w565 -> [_ w574]
              frame #0 {
                n572 = call-poly "AO Update Channel (scaled value).vi"("value"=sgl 0.0, "channel (0)"=w571, "device"=w572) -> ()
              }
              frame #1 {
                n573 = call-poly "AO Update Channel (scaled value).vi"("value"=w574, "channel (0)"=w576, "device"=w575) -> ()
              }
            }
          }
          event #31 {
            n574 = event-data() -> ()  [unwired: 1 in, 6 out]
            n575 = call "AOTFSettings.vi"() -> ("AOTF Setting (Output)"=w582:T15)  [unwired: 2 in]
            n576 = call "AnalogSettings.vi"() -> ("Analog Settings (output)"=w581:T14)  [unwired: 2 in]
            n577 = Unbundle By Name(w582) -> ("Laser 2 Output Channel"=w579:tag, "AOTF  2 Output Voltage"=w578:dbl)
            n578 = Unbundle By Name(w581) -> ("PCI 671x Device Number"=w580:u32)
            n579 = case shown="False" "Laser 2" {
              tunnel: w580 -> [w584 w587]
              tunnel: w579 -> [w583 w588]
              tunnel: w578 -> [_ w586]
              frame #0 {
                n580 = call-poly "AO Update Channel (scaled value).vi"("value"=sgl 0.0, "channel (0)"=w583, "device"=w584) -> ()
              }
              frame #1 {
                n581 = call-poly "AO Update Channel (scaled value).vi"("value"=w586, "channel (0)"=w588, "device"=w587) -> ()
              }
            }
          }
          event #32 {
            n582 = event-data() -> ()  [unwired: 1 in, 6 out]
            n583 = call "AnalogSettings.vi"() -> ("Analog Settings (output)"=w593:T14)  [unwired: 2 in]
            n584 = call "AOTFSettings.vi"() -> ("AOTF Setting (Output)"=w594:T15)  [unwired: 2 in]
            n585 = Unbundle By Name(w594) -> ("Laser 3 Output Channel"=w591:tag, "AOTF  3 Output Voltage"=w590:dbl)
            n586 = Unbundle By Name(w593) -> ("PCI 671x Device Number"=w592:u32)
            n587 = case shown="True" "Laser 3" {
              tunnel: w592 -> [w596 w599]
              tunnel: w591 -> [w595 w600]
              tunnel: w590 -> [_ w598]
              frame #0 {
                n588 = call-poly "AO Update Channel (scaled value).vi"("value"=sgl 0.0, "channel (0)"=w595, "device"=w596) -> ()
              }
              frame #1 {
                n589 = call-poly "AO Update Channel (scaled value).vi"("value"=w598, "channel (0)"=w600, "device"=w599) -> ()
              }
            }
          }
          event #33 {
            n590 = event-data() -> ()  [unwired: 1 in, 6 out]
            n591 = call "AOTFSettings.vi"() -> ("AOTF Setting (Output)"=w606:T15)  [unwired: 2 in]
            n592 = call "AnalogSettings.vi"() -> ("Analog Settings (output)"=w605:T14)  [unwired: 2 in]
            n593 = Unbundle By Name(w606) -> ("Laser 4 Output Channel"=w603:tag, "AOTF  4 Output Voltage"=w602:dbl)
            n594 = Unbundle By Name(w605) -> ("PCI 671x Device Number"=w604:u32)
            n595 = case shown="True" "Laser 4" {
              tunnel: w604 -> [w608 w611]
              tunnel: w603 -> [w607 w612]
              tunnel: w602 -> [_ w610]
              frame #0 {
                n596 = call-poly "AO Update Channel (scaled value).vi"("value"=sgl 0.0, "channel (0)"=w607, "device"=w608) -> ()
              }
              frame #1 {
                n597 = call-poly "AO Update Channel (scaled value).vi"("value"=w610, "channel (0)"=w612, "device"=w611) -> ()
              }
            }
          }
        }
      }
    }
  }
